vi "SLSC Create Tree Control from EDS datatype.vi"(7 "Property Tree":refnum<vi>, 8 "error in (no error)":errorcluster, 9 "Channel Values":dbl[](array[numeric]), 10 "Properties to enable":string[](array[string]), 11 "SLSC EDS module":T4={"vendorNum"=4660, "vendorName"="National Instruments", "vendorPrefix"="NI", "productNum"=4098, "productName"="SLSC-12201", "capsVersion"="1.0.0a9", "capsSpecVersion"=2, "capsSpecOldestCompatibleVersion"=2, "enums"=[{"name"="NI.Line.Direction", "description-en"="Enumerated values for the direction and output type of a DIO line", "values"=[{"name"="Input", "description-en"="Route line from the front I/O connector to the rear I/O connector", "value"=0}, {"name"="Output_Source", "description-en"="Route line from the rear I/O connector to the front I/O connector with sourcing output topology", "value"=1}, {"name"="Output_Sink", "description-en"="Route line from the rear I/O connector to the front I/O connector with sinking output topology", "value"=2}, {"name"="Output_PushPull", "description-en"="Route line from the rear I/O connector to the front I/O connector with push-pull output topology", "value"=3}]}, {"name"="NI.VsupSource", "description-en"="Enumerated values for the selection of the bank's voltage source", "values"=[{"name"="Vsup_Off", "description-en"="Select neither supply voltage", "value"=0}, {"name"="Vsup_0", "description-en"="Select supply voltage 0", "value"=1}, {"name"="Vsup_1", "description-en"="Select supply voltage 1", "value"=2}]}], "properties"=[{"name"="NI.ModuleControllerVersion", "bitfield"="RevisionReg/DateCode", "value"=variant, "dataType"="UInt32", "min"=variant, "max"=variant, "scale"="", "access"=""}, {"name"="NI.RearBufferState", "bitfield"="RearIOConnectorChannelStateReg/ChannelState", "value"=variant, "dataType"="UInt32", "min"=variant, "max"=variant, "scale"="", "access"=""}, {"name"="NI.FrontBufferState", "bitfield"="FrontIOConnectorChannelStateReg/ChannelState", "value"=variant, "dataType"="UInt32", "min"=variant, "max"=variant, "scale"="", "access"=""}, {"name"="NI.Status24VPowerFailed", "bitfield"="ModuleStatusReg/Status24V_PowerFailed", "value"=variant, "dataType"="Bool", "min"=variant, "max"=variant, "scale"="", "access"=""}, {"name"="NI.Status24VPowerGood", "bitfield"="ModuleStatusReg/Status24V_PowerGood", "value"=variant, "dataType"="Bool", "min"=variant, "max"=variant, "scale"="", "access"=""}, {"name"="NI.Status3_3VPowerGood", "bitfield"="ModuleStatusReg/Status3_3V_PowerGood", "value"=variant, "dataType"="Bool", "min"=variant, "max"=variant, "scale"="", "access"=""}, {"name"="NI.TestModeEnable", "bitfield"="TestModeEnableReg/TestModeEnable", "value"=variant, "dataType"="Bool", "min"=variant, "max"=variant, "scale"="", "access"=""}, {"name"="NI.TestModeValue", "bitfield"="TestModeValueReg/TestModeValue", "value"=variant, "dataType"="UInt32", "min"=variant, "max"=variant, "scale"="", "access"=""}], "commands"=[{"name"="NI.UpdateChannelConfiguration", "description-en"="Command to complete updating physical channel properties", "documentation-en"="This command enables simultaneous updating of the functional state of the module's physical channel configuration. Simultaneous updating of the physical channels' properties prevents the register write commit order from creating unexpected channel configuration states. Run this command to make changes to physical channels' properties take effect.", "startBitfield"="ConfigCommandReg/ChannelConfigurationUpdate", "waitTimeInMs"=5, "doneBitfield"="", "doneInterrupt"="", "doneTimeoutInMs"=0, "value"=variant}, {"name"="NI.UpdateTestMode", "description-en"="Command to complete updating Test Mode properties", "documentation-en"="This command enable simultaneous updating of the functional state of the module's Test Mode configuration. Run this command to make changes to Test Mode properties take effect.", "startBitfield"="ConfigCommandReg/TestModeUpdate", "waitTimeInMs"=0, "doneBitfield"="", "doneInterrupt"="", "doneTimeoutInMs"=0, "value"=variant}, {"name"="NI.Acknowledge24VPowerFailed", "description-en"="Command to acknowledge a latched 24V power failure status", "documentation-en"="This command tries to clear the module's latched true state for the NI.Status24V_PowerFailed property. This command will have no effect on the latched state if the NI.Status24V_PowerGood property is still false.", "startBitfield"="ModuleStatusReg/Status24V_PowerFailedAck", "waitTimeInMs"=0, "doneBitfield"="", "doneInterrupt"="", "doneTimeoutInMs"=0, "value"=variant}], "scales"=[{"name"="InputThreshold33V_Scale", "description-en"="Scales a given voltage into the 10-bit threshold value for the 33V input range", "m"=0.02335, "b"=3.706, "forwardCoeffs"=[], "reverseCoeffs"=[], "coercion"="", "table"=[]}, {"name"="InputThreshold5V_Scale", "description-en"="Scales a given voltage into the 10-bit threshold value for the 5V input range", "m"=0.00441, "b"=0.7, "forwardCoeffs"=[], "reverseCoeffs"=[], "coercion"="", "table"=[]}], "physicalChannels"=[{"name"="bank0", "description-en"="Bank of digital input/output lines on connector J1", "commands"=[], "properties"=[{"name"="NI.VsupSelect", "bitfield"="BankConfigurationReg/Bank0_VsupSelect", "value"=variant, "dataType"="NI.VsupSource", "min"=variant, "max"=variant, "scale"="", "access"=""}, {"name"="NI.RangeEnable5V", "bitfield"="BankConfigurationReg/Bank0_RangeEnable5V", "value"=variant, "dataType"="Bool", "min"=variant, "max"=variant, "scale"="", "access"=""}, {"name"="NI.InputThreshold5V", "bitfield"="BankConfigurationReg/Bank0_InputThreshold5V", "value"=variant, "dataType"="Double", "min"=variant(ext 0.74), "max"=variant(ext 5.1999999999999999998), "scale"="InputThreshold5V_Scale", "access"=""}, {"name"="NI.InputThreshold33V", "bitfield"="BankConfigurationReg/Bank0_InputThreshold33V", "value"=variant, "dataType"="Double", "min"=variant(ext 4.0), "max"=variant(ext 27.7), "scale"="InputThreshold33V_Scale", "access"=""}]}, {"name"="bank1", "description-en"="Bank of digital input/output lines on connector J2", "commands"=[], "properties"=[{"name"="NI.VsupSelect", "bitfield"="BankConfigurationReg/Bank1_VsupSelect", "value"=variant, "dataType"="NI.VsupSource", "min"=variant, "max"=variant, "scale"="", "access"=""}, {"name"="NI.RangeEnable5V", "bitfield"="BankConfigurationReg/Bank1_RangeEnable5V", "value"=variant, "dataType"="Bool", "min"=variant, "max"=variant, "scale"="", "access"=""}, {"name"="NI.InputThreshold5V", "bitfield"="BankConfigurationReg/Bank1_InputThreshold5V", "value"=variant, "dataType"="Double", "min"=variant(ext 0.74), "max"=variant(ext 5.1999999999999999998), "scale"="InputThreshold5V_Scale", "access"=""}, {"name"="NI.InputThreshold33V", "bitfield"="BankConfigurationReg/Bank1_InputThreshold33V", "value"=variant, "dataType"="Double", "min"=variant(ext 4.0), "max"=variant(ext 27.7), "scale"="InputThreshold33V_Scale", "access"=""}]}, {"name"="port0/line0", "description-en"="Configurable digital input/output line with index 0 in bank0.", "commands"=[], "properties"=[{"name"="NI.Line.Index", "bitfield"="", "value"=variant(u64 0), "dataType"="UInt32", "min"=variant, "max"=variant, "scale"="", "access"=""}, {"name"="NI.Line.Direction", "bitfield"="ChannelDirectionReg/Port0_Line0_Direction", "value"=variant, "dataType"="NI.Line.Direction", "min"=variant, "max"=variant, "scale"="", "access"=""}, {"name"="NI.Line.Enable", "bitfield"="ChannelEnableReg/Port0_Line0_Enable", "value"=variant, "dataType"="Bool", "min"=variant, "max"=variant, "scale"="", "access"=""}]}, {"name"="port0/line1", "description-en"="Configurable digital input/output line with index 1 in bank0.", "commands"=[], "properties"=[{"name"="NI.Line.Index", "bitfield"="", "value"=variant(u64 1), "dataType"="UInt32", "min"=variant, "max"=variant, "scale"="", "access"=""}, {"name"="NI.Line.Direction", "bitfield"="ChannelDirectionReg/Port0_Line1_Direction", "value"=variant, "dataType"="NI.Line.Direction", "min"=variant, "max"=variant, "scale"="", "access"=""}, {"name"="NI.Line.Enable", "bitfield"="ChannelEnableReg/Port0_Line1_Enable", "value"=variant, "dataType"="Bool", "min"=variant, "max"=variant, "scale"="", "access"=""}]}, {"name"="port0/line2", "description-en"="Configurable digital input/output line with index 2 in bank0.", "commands"=[], "properties"=[{"name"="NI.Line.Index", "bitfield"="", "value"=variant(u64 2), "dataType"="UInt32", "min"=variant, "max"=variant, "scale"="", "access"=""}, {"name"="NI.Line.Direction", "bitfield"="ChannelDirectionReg/Port0_Line2_Direction", "value"=variant, "dataType"="NI.Line.Direction", "min"=variant, "max"=variant, "scale"="", "access"=""}, {"name"="NI.Line.Enable", "bitfield"="ChannelEnableReg/Port0_Line2_Enable", "value"=variant, "dataType"="Bool", "min"=variant, "max"=variant, "scale"="", "access"=""}]}, {"name"="port0/line3", "description-en"="Configurable digital input/output line with index 3 in bank0.", "commands"=[], "properties"=[{"name"="NI.Line.Index", "bitfield"="", "value"=variant(u64 3), "dataType"="UInt32", "min"=variant, "max"=variant, "scale"="", "access"=""}, {"name"="NI.Line.Direction", "bitfield"="ChannelDirectionReg/Port0_Line3_Direction", "value"=variant, "dataType"="NI.Line.Direction", "min"=variant, "max"=variant, "scale"="", "access"=""}, {"name"="NI.Line.Enable", "bitfield"="ChannelEnableReg/Port0_Line3_Enable", "value"=variant, "dataType"="Bool", "min"=variant, "max"=variant, "scale"="", "access"=""}]}, {"name"="port0/line4", "description-en"="Configurable digital input/output line with index 4 in bank0.", "commands"=[], "properties"=[{"name"="NI.Line.Index", "bitfield"="", "value"=variant(u64 4), "dataType"="UInt32", "min"=variant, "max"=variant, "scale"="", "access"=""}, {"name"="NI.Line.Direction", "bitfield"="ChannelDirectionReg/Port0_Line4_Direction", "value"=variant, "dataType"="NI.Line.Direction", "min"=variant, "max"=variant, "scale"="", "access"=""}, {"name"="NI.Line.Enable", "bitfield"="ChannelEnableReg/Port0_Line4_Enable", "value"=variant, "dataType"="Bool", "min"=variant, "max"=variant, "scale"="", "access"=""}]}, {"name"="port0/line5", "description-en"="Configurable digital input/output line with index 5 in bank0.", "commands"=[], "properties"=[{"name"="NI.Line.Index", "bitfield"="", "value"=variant(u64 5), "dataType"="UInt32", "min"=variant, "max"=variant, "scale"="", "access"=""}, {"name"="NI.Line.Direction", "bitfield"="ChannelDirectionReg/Port0_Line5_Direction", "value"=variant, "dataType"="NI.Line.Direction", "min"=variant, "max"=variant, "scale"="", "access"=""}, {"name"="NI.Line.Enable", "bitfield"="ChannelEnableReg/Port0_Line5_Enable", "value"=variant, "dataType"="Bool", "min"=variant, "max"=variant, "scale"="", "access"=""}]}, {"name"="port0/line6", "description-en"="Configurable digital input/output line with index 6 in bank0.", "commands"=[], "properties"=[{"name"="NI.Line.Index", "bitfield"="", "value"=variant(u64 6), "dataType"="UInt32", "min"=variant, "max"=variant, "scale"="", "access"=""}, {"name"="NI.Line.Direction", "bitfield"="ChannelDirectionReg/Port0_Line6_Direction", "value"=variant, "dataType"="NI.Line.Direction", "min"=variant, "max"=variant, "scale"="", "access"=""}, {"name"="NI.Line.Enable", "bitfield"="ChannelEnableReg/Port0_Line6_Enable", "value"=variant, "dataType"="Bool", "min"=variant, "max"=variant, "scale"="", "access"=""}]}, {"name"="port0/line7", "description-en"="Configurable digital input/output line with index 7 in bank0.", "commands"=[], "properties"=[{"name"="NI.Line.Index", "bitfield"="", "value"=variant(u64 7), "dataType"="UInt32", "min"=variant, "max"=variant, "scale"="", "access"=""}, {"name"="NI.Line.Direction", "bitfield"="ChannelDirectionReg/Port0_Line7_Direction", "value"=variant, "dataType"="NI.Line.Direction", "min"=variant, "max"=variant, "scale"="", "access"=""}, {"name"="NI.Line.Enable", "bitfield"="ChannelEnableReg/Port0_Line7_Enable", "value"=variant, "dataType"="Bool", "min"=variant, "max"=variant, "scale"="", "access"=""}]}, {"name"="port1/line0", "description-en"="Configurable digital input/output line with index 8 in bank0.", "commands"=[], "properties"=[{"name"="NI.Line.Index", "bitfield"="", "value"=variant(u64 8), "dataType"="UInt32", "min"=variant, "max"=variant, "scale"="", "access"=""}, {"name"="NI.Line.Direction", "bitfield"="ChannelDirectionReg/Port1_Line0_Direction", "value"=variant, "dataType"="NI.Line.Direction", "min"=variant, "max"=variant, "scale"="", "access"=""}, {"name"="NI.Line.Enable", "bitfield"="ChannelEnableReg/Port1_Line0_Enable", "value"=variant, "dataType"="Bool", "min"=variant, "max"=variant, "scale"="", "access"=""}]}, {"name"="port1/line1", "description-en"="Configurable digital input/output line with index 9 in bank0.", "commands"=[], "properties"=[{"name"="NI.Line.Index", "bitfield"="", "value"=variant(u64 9), "dataType"="UInt32", "min"=variant, "max"=variant, "scale"="", "access"=""}, {"name"="NI.Line.Direction", "bitfield"="ChannelDirectionReg/Port1_Line1_Direction", "value"=variant, "dataType"="NI.Line.Direction", "min"=variant, "max"=variant, "scale"="", "access"=""}, {"name"="NI.Line.Enable", "bitfield"="ChannelEnableReg/Port1_Line1_Enable", "value"=variant, "dataType"="Bool", "min"=variant, "max"=variant, "scale"="", "access"=""}]}, {"name"="port1/line2", "description-en"="Configurable digital input/output line with index 10 in bank0.", "commands"=[], "properties"=[{"name"="NI.Line.Index", "bitfield"="", "value"=variant(u64 10), "dataType"="UInt32", "min"=variant, "max"=variant, "scale"="", "access"=""}, {"name"="NI.Line.Direction", "bitfield"="ChannelDirectionReg/Port1_Line2_Direction", "value"=variant, "dataType"="NI.Line.Direction", "min"=variant, "max"=variant, "scale"="", "access"=""}, {"name"="NI.Line.Enable", "bitfield"="ChannelEnableReg/Port1_Line2_Enable", "value"=variant, "dataType"="Bool", "min"=variant, "max"=variant, "scale"="", "access"=""}]}, {"name"="port1/line3", "description-en"="Configurable digital input/output line with index 11 in bank0.", "commands"=[], "properties"=[{"name"="NI.Line.Index", "bitfield"="", "value"=variant(u64 11), "dataType"="UInt32", "min"=variant, "max"=variant, "scale"="", "access"=""}, {"name"="NI.Line.Direction", "bitfield"="ChannelDirectionReg/Port1_Line3_Direction", "value"=variant, "dataType"="NI.Line.Direction", "min"=variant, "max"=variant, "scale"="", "access"=""}, {"name"="NI.Line.Enable", "bitfield"="ChannelEnableReg/Port1_Line3_Enable", "value"=variant, "dataType"="Bool", "min"=variant, "max"=variant, "scale"="", "access"=""}]}, {"name"="port1/line4", "description-en"="Configurable digital input/output line with index 12 in bank0.", "commands"=[], "properties"=[{"name"="NI.Line.Index", "bitfield"="", "value"=variant(u64 12), "dataType"="UInt32", "min"=variant, "max"=variant, "scale"="", "access"=""}, {"name"="NI.Line.Direction", "bitfield"="ChannelDirectionReg/Port1_Line4_Direction", "value"=variant, "dataType"="NI.Line.Direction", "min"=variant, "max"=variant, "scale"="", "access"=""}, {"name"="NI.Line.Enable", "bitfield"="ChannelEnableReg/Port1_Line4_Enable", "value"=variant, "dataType"="Bool", "min"=variant, "max"=variant, "scale"="", "access"=""}]}, {"name"="port1/line5", "description-en"="Configurable digital input/output line with index 13 in bank0.", "commands"=[], "properties"=[{"name"="NI.Line.Index", "bitfield"="", "value"=variant(u64 13), "dataType"="UInt32", "min"=variant, "max"=variant, "scale"="", "access"=""}, {"name"="NI.Line.Direction", "bitfield"="ChannelDirectionReg/Port1_Line5_Direction", "value"=variant, "dataType"="NI.Line.Direction", "min"=variant, "max"=variant, "scale"="", "access"=""}, {"name"="NI.Line.Enable", "bitfield"="ChannelEnableReg/Port1_Line5_Enable", "value"=variant, "dataType"="Bool", "min"=variant, "max"=variant, "scale"="", "access"=""}]}, {"name"="port1/line6", "description-en"="Configurable digital input/output line with index 14 in bank0.", "commands"=[], "properties"=[{"name"="NI.Line.Index", "bitfield"="", "value"=variant(u64 14), "dataType"="UInt32", "min"=variant, "max"=variant, "scale"="", "access"=""}, {"name"="NI.Line.Direction", "bitfield"="ChannelDirectionReg/Port1_Line6_Direction", "value"=variant, "dataType"="NI.Line.Direction", "min"=variant, "max"=variant, "scale"="", "access"=""}, {"name"="NI.Line.Enable", "bitfield"="ChannelEnableReg/Port1_Line6_Enable", "value"=variant, "dataType"="Bool", "min"=variant, "max"=variant, "scale"="", "access"=""}]}, {"name"="port1/line7", "description-en"="Configurable digital input/output line with index 15 in bank0.", "commands"=[], "properties"=[{"name"="NI.Line.Index", "bitfield"="", "value"=variant(u64 15), "dataType"="UInt32", "min"=variant, "max"=variant, "scale"="", "access"=""}, {"name"="NI.Line.Direction", "bitfield"="ChannelDirectionReg/Port1_Line7_Direction", "value"=variant, "dataType"="NI.Line.Direction", "min"=variant, "max"=variant, "scale"="", "access"=""}, {"name"="NI.Line.Enable", "bitfield"="ChannelEnableReg/Port1_Line7_Enable", "value"=variant, "dataType"="Bool", "min"=variant, "max"=variant, "scale"="", "access"=""}]}, {"name"="port2/line0", "description-en"="Configurable digital input/output line with index 16 in bank1.", "commands"=[], "properties"=[{"name"="NI.Line.Index", "bitfield"="", "value"=variant(u64 16), "dataType"="UInt32", "min"=variant, "max"=variant, "scale"="", "access"=""}, {"name"="NI.Line.Direction", "bitfield"="ChannelDirectionReg/Port2_Line0_Direction", "value"=variant, "dataType"="NI.Line.Direction", "min"=variant, "max"=variant, "scale"="", "access"=""}, {"name"="NI.Line.Enable", "bitfield"="ChannelEnableReg/Port2_Line0_Enable", "value"=variant, "dataType"="Bool", "min"=variant, "max"=variant, "scale"="", "access"=""}]}, {"name"="port2/line1", "description-en"="Configurable digital input/output line with index 17 in bank1.", "commands"=[], "properties"=[{"name"="NI.Line.Index", "bitfield"="", "value"=variant(u64 17), "dataType"="UInt32", "min"=variant, "max"=variant, "scale"="", "access"=""}, {"name"="NI.Line.Direction", "bitfield"="ChannelDirectionReg/Port2_Line1_Direction", "value"=variant, "dataType"="NI.Line.Direction", "min"=variant, "max"=variant, "scale"="", "access"=""}, {"name"="NI.Line.Enable", "bitfield"="ChannelEnableReg/Port2_Line1_Enable", "value"=variant, "dataType"="Bool", "min"=variant, "max"=variant, "scale"="", "access"=""}]}, {"name"="port2/line2", "description-en"="Configurable digital input/output line with index 18 in bank1.", "commands"=[], "properties"=[{"name"="NI.Line.Index", "bitfield"="", "value"=variant(u64 18), "dataType"="UInt32", "min"=variant, "max"=variant, "scale"="", "access"=""}, {"name"="NI.Line.Direction", "bitfield"="ChannelDirectionReg/Port2_Line2_Direction", "value"=variant, "dataType"="NI.Line.Direction", "min"=variant, "max"=variant, "scale"="", "access"=""}, {"name"="NI.Line.Enable", "bitfield"="ChannelEnableReg/Port2_Line2_Enable", "value"=variant, "dataType"="Bool", "min"=variant, "max"=variant, "scale"="", "access"=""}]}, {"name"="port2/line3", "description-en"="Configurable digital input/output line with index 19 in bank1.", "commands"=[], "properties"=[{"name"="NI.Line.Index", "bitfield"="", "value"=variant(u64 19), "dataType"="UInt32", "min"=variant, "max"=variant, "scale"="", "access"=""}, {"name"="NI.Line.Direction", "bitfield"="ChannelDirectionReg/Port2_Line3_Direction", "value"=variant, "dataType"="NI.Line.Direction", "min"=variant, "max"=variant, "scale"="", "access"=""}, {"name"="NI.Line.Enable", "bitfield"="ChannelEnableReg/Port2_Line3_Enable", "value"=variant, "dataType"="Bool", "min"=variant, "max"=variant, "scale"="", "access"=""}]}, {"name"="port2/line4", "description-en"="Configurable digital input/output line with index 20 in bank1.", "commands"=[], "properties"=[{"name"="NI.Line.Index", "bitfield"="", "value"=variant(u64 20), "dataType"="UInt32", "min"=variant, "max"=variant, "scale"="", "access"=""}, {"name"="NI.Line.Direction", "bitfield"="ChannelDirectionReg/Port2_Line4_Direction", "value"=variant, "dataType"="NI.Line.Direction", "min"=variant, "max"=variant, "scale"="", "access"=""}, {"name"="NI.Line.Enable", "bitfield"="ChannelEnableReg/Port2_Line4_Enable", "value"=variant, "dataType"="Bool", "min"=variant, "max"=variant, "scale"="", "access"=""}]}, {"name"="port2/line5", "description-en"="Configurable digital input/output line with index 21 in bank1.", "commands"=[], "properties"=[{"name"="NI.Line.Index", "bitfield"="", "value"=variant(u64 21), "dataType"="UInt32", "min"=variant, "max"=variant, "scale"="", "access"=""}, {"name"="NI.Line.Direction", "bitfield"="ChannelDirectionReg/Port2_Line5_Direction", "value"=variant, "dataType"="NI.Line.Direction", "min"=variant, "max"=variant, "scale"="", "access"=""}, {"name"="NI.Line.Enable", "bitfield"="ChannelEnableReg/Port2_Line5_Enable", "value"=variant, "dataType"="Bool", "min"=variant, "max"=variant, "scale"="", "access"=""}]}, {"name"="port2/line6", "description-en"="Configurable digital input/output line with index 22 in bank1.", "commands"=[], "properties"=[{"name"="NI.Line.Index", "bitfield"="", "value"=variant(u64 22), "dataType"="UInt32", "min"=variant, "max"=variant, "scale"="", "access"=""}, {"name"="NI.Line.Direction", "bitfield"="ChannelDirectionReg/Port2_Line6_Direction", "value"=variant, "dataType"="NI.Line.Direction", "min"=variant, "max"=variant, "scale"="", "access"=""}, {"name"="NI.Line.Enable", "bitfield"="ChannelEnableReg/Port2_Line6_Enable", "value"=variant, "dataType"="Bool", "min"=variant, "max"=variant, "scale"="", "access"=""}]}, {"name"="port2/line7", "description-en"="Configurable digital input/output line with index 23 in bank1.", "commands"=[], "properties"=[{"name"="NI.Line.Index", "bitfield"="", "value"=variant(u64 23), "dataType"="UInt32", "min"=variant, "max"=variant, "scale"="", "access"=""}, {"name"="NI.Line.Direction", "bitfield"="ChannelDirectionReg/Port2_Line7_Direction", "value"=variant, "dataType"="NI.Line.Direction", "min"=variant, "max"=variant, "scale"="", "access"=""}, {"name"="NI.Line.Enable", "bitfield"="ChannelEnableReg/Port2_Line7_Enable", "value"=variant, "dataType"="Bool", "min"=variant, "max"=variant, "scale"="", "access"=""}]}, {"name"="port3/line0", "description-en"="Configurable digital input/output line with index 24 in bank1.", "commands"=[], "properties"=[{"name"="NI.Line.Index", "bitfield"="", "value"=variant(u64 24), "dataType"="UInt32", "min"=variant, "max"=variant, "scale"="", "access"=""}, {"name"="NI.Line.Direction", "bitfield"="ChannelDirectionReg/Port3_Line0_Direction", "value"=variant, "dataType"="NI.Line.Direction", "min"=variant, "max"=variant, "scale"="", "access"=""}, {"name"="NI.Line.Enable", "bitfield"="ChannelEnableReg/Port3_Line0_Enable", "value"=variant, "dataType"="Bool", "min"=variant, "max"=variant, "scale"="", "access"=""}]}, {"name"="port3/line1", "description-en"="Configurable digital input/output line with index 25 in bank1.", "commands"=[], "properties"=[{"name"="NI.Line.Index", "bitfield"="", "value"=variant(u64 25), "dataType"="UInt32", "min"=variant, "max"=variant, "scale"="", "access"=""}, {"name"="NI.Line.Direction", "bitfield"="ChannelDirectionReg/Port3_Line1_Direction", "value"=variant, "dataType"="NI.Line.Direction", "min"=variant, "max"=variant, "scale"="", "access"=""}, {"name"="NI.Line.Enable", "bitfield"="ChannelEnableReg/Port3_Line1_Enable", "value"=variant, "dataType"="Bool", "min"=variant, "max"=variant, "scale"="", "access"=""}]}, {"name"="port3/line2", "description-en"="Configurable digital input/output line with index 26 in bank1.", "commands"=[], "properties"=[{"name"="NI.Line.Index", "bitfield"="", "value"=variant(u64 26), "dataType"="UInt32", "min"=variant, "max"=variant, "scale"="", "access"=""}, {"name"="NI.Line.Direction", "bitfield"="ChannelDirectionReg/Port3_Line2_Direction", "value"=variant, "dataType"="NI.Line.Direction", "min"=variant, "max"=variant, "scale"="", "access"=""}, {"name"="NI.Line.Enable", "bitfield"="ChannelEnableReg/Port3_Line2_Enable", "value"=variant, "dataType"="Bool", "min"=variant, "max"=variant, "scale"="", "access"=""}]}, {"name"="port3/line3", "description-en"="Configurable digital input/output line with index 27 in bank1.", "commands"=[], "properties"=[{"name"="NI.Line.Index", "bitfield"="", "value"=variant(u64 27), "dataType"="UInt32", "min"=variant, "max"=variant, "scale"="", "access"=""}, {"name"="NI.Line.Direction", "bitfield"="ChannelDirectionReg/Port3_Line3_Direction", "value"=variant, "dataType"="NI.Line.Direction", "min"=variant, "max"=variant, "scale"="", "access"=""}, {"name"="NI.Line.Enable", "bitfield"="ChannelEnableReg/Port3_Line3_Enable", "value"=variant, "dataType"="Bool", "min"=variant, "max"=variant, "scale"="", "access"=""}]}, {"name"="port3/line4", "description-en"="Configurable digital input/output line with index 28 in bank1.", "commands"=[], "properties"=[{"name"="NI.Line.Index", "bitfield"="", "value"=variant(u64 28), "dataType"="UInt32", "min"=variant, "max"=variant, "scale"="", "access"=""}, {"name"="NI.Line.Direction", "bitfield"="ChannelDirectionReg/Port3_Line4_Direction", "value"=variant, "dataType"="NI.Line.Direction", "min"=variant, "max"=variant, "scale"="", "access"=""}, {"name"="NI.Line.Enable", "bitfield"="ChannelEnableReg/Port3_Line4_Enable", "value"=variant, "dataType"="Bool", "min"=variant, "max"=variant, "scale"="", "access"=""}]}, {"name"="port3/line5", "description-en"="Configurable digital input/output line with index 29 in bank1.", "commands"=[], "properties"=[{"name"="NI.Line.Index", "bitfield"="", "value"=variant(u64 29), "dataType"="UInt32", "min"=variant, "max"=variant, "scale"="", "access"=""}, {"name"="NI.Line.Direction", "bitfield"="ChannelDirectionReg/Port3_Line5_Direction", "value"=variant, "dataType"="NI.Line.Direction", "min"=variant, "max"=variant, "scale"="", "access"=""}, {"name"="NI.Line.Enable", "bitfield"="ChannelEnableReg/Port3_Line5_Enable", "value"=variant, "dataType"="Bool", "min"=variant, "max"=variant, "scale"="", "access"=""}]}, {"name"="port3/line6", "description-en"="Configurable digital input/output line with index 30 in bank1.", "commands"=[], "properties"=[{"name"="NI.Line.Index", "bitfield"="", "value"=variant(u64 30), "dataType"="UInt32", "min"=variant, "max"=variant, "scale"="", "access"=""}, {"name"="NI.Line.Direction", "bitfield"="ChannelDirectionReg/Port3_Line6_Direction", "value"=variant, "dataType"="NI.Line.Direction", "min"=variant, "max"=variant, "scale"="", "access"=""}, {"name"="NI.Line.Enable", "bitfield"="ChannelEnableReg/Port3_Line6_Enable", "value"=variant, "dataType"="Bool", "min"=variant, "max"=variant, "scale"="", "access"=""}]}, {"name"="port3/line7", "description-en"="Configurable digital input/output line with index 31 in bank1.", "commands"=[], "properties"=[{"name"="NI.Line.Index", "bitfield"="", "value"=variant(u64 31), "dataType"="UInt32", "min"=variant, "max"=variant, "scale"="", "access"=""}, {"name"="NI.Line.Direction", "bitfield"="ChannelDirectionReg/Port3_Line7_Direction", "value"=variant, "dataType"="NI.Line.Direction", "min"=variant, "max"=variant, "scale"="", "access"=""}, {"name"="NI.Line.Enable", "bitfield"="ChannelEnableReg/Port3_Line7_Enable", "value"=variant, "dataType"="Bool", "min"=variant, "max"=variant, "scale"="", "access"=""}]}], "registerMap"={"registers"=[{"name"="RevisionReg", "description-en"="Register for the DateCode", "access"="ReadOnly", "address"=0, "size"=32, "bitfields"=[{"name"="DateCode", "description-en"="CPLD revision date code", "offset"=0, "size"=32, "signed"=FALSE, "strobe"=FALSE}]}, {"name"="RearIOConnectorChannelStateReg", "description-en"="Register for the rear I/O connector channel state", "access"="ReadOnly", "address"=4, "size"=32, "bitfields"=[{"name"="ChannelState", "description-en"="Logic state of all rear I/O connector input buffers", "offset"=0, "size"=32, "signed"=FALSE, "strobe"=FALSE}]}, {"name"="FrontIOConnectorChannelStateReg", "description-en"="Register for the front I/O connector channel state", "access"="ReadOnly", "address"=8, "size"=32, "bitfields"=[{"name"="ChannelState", "description-en"="Logic state of all front I/O connector input buffers", "offset"=0, "size"=32, "signed"=FALSE, "strobe"=FALSE}]}, {"name"="ModuleStatusReg", "description-en"="Register for monitoring board-level module status", "access"="ReadWrite", "address"=12, "size"=8, "bitfields"=[{"name"="Status3_3V_PowerGood", "description-en"="3.3V power status (always '1' on successful module access)", "offset"=0, "size"=1, "signed"=FALSE, "strobe"=FALSE}, {"name"="Status24V_PowerGood", "description-en"="24V power status", "offset"=1, "size"=1, "signed"=FALSE, "strobe"=FALSE}, {"name"="Status24V_PowerFailed", "description-en"="Latching status indicating 24V power failure", "offset"=2, "size"=1, "signed"=FALSE, "strobe"=FALSE}, {"name"="Status24V_PowerFailedAck", "description-en"="Target bitfield for the NI.Status24V_PowerFailedAck command", "offset"=3, "size"=1, "signed"=FALSE, "strobe"=TRUE}]}, {"name"="ChannelDirectionReg", "description-en"="Register for setting channel direction (This register requires having a valid \"initalValue\" set.)", "access"="ReadWrite", "address"=64, "size"=64, "bitfields"=[{"name"="Port0_Line0_Direction", "description-en"="", "offset"=0, "size"=2, "signed"=FALSE, "strobe"=FALSE}, {"name"="Port0_Line1_Direction", "description-en"="", "offset"=2, "size"=2, "signed"=FALSE, "strobe"=FALSE}, {"name"="Port0_Line2_Direction", "description-en"="", "offset"=4, "size"=2, "signed"=FALSE, "strobe"=FALSE}, {"name"="Port0_Line3_Direction", "description-en"="", "offset"=6, "size"=2, "signed"=FALSE, "strobe"=FALSE}, {"name"="Port0_Line4_Direction", "description-en"="", "offset"=8, "size"=2, "signed"=FALSE, "strobe"=FALSE}, {"name"="Port0_Line5_Direction", "description-en"="", "offset"=10, "size"=2, "signed"=FALSE, "strobe"=FALSE}, {"name"="Port0_Line6_Direction", "description-en"="", "offset"=12, "size"=2, "signed"=FALSE, "strobe"=FALSE}, {"name"="Port0_Line7_Direction", "description-en"="", "offset"=14, "size"=2, "signed"=FALSE, "strobe"=FALSE}, {"name"="Port1_Line0_Direction", "description-en"="", "offset"=16, "size"=2, "signed"=FALSE, "strobe"=FALSE}, {"name"="Port1_Line1_Direction", "description-en"="", "offset"=18, "size"=2, "signed"=FALSE, "strobe"=FALSE}, {"name"="Port1_Line2_Direction", "description-en"="", "offset"=20, "size"=2, "signed"=FALSE, "strobe"=FALSE}, {"name"="Port1_Line3_Direction", "description-en"="", "offset"=22, "size"=2, "signed"=FALSE, "strobe"=FALSE}, {"name"="Port1_Line4_Direction", "description-en"="", "offset"=24, "size"=2, "signed"=FALSE, "strobe"=FALSE}, {"name"="Port1_Line5_Direction", "description-en"="", "offset"=26, "size"=2, "signed"=FALSE, "strobe"=FALSE}, {"name"="Port1_Line6_Direction", "description-en"="", "offset"=28, "size"=2, "signed"=FALSE, "strobe"=FALSE}, {"name"="Port1_Line7_Direction", "description-en"="", "offset"=30, "size"=2, "signed"=FALSE, "strobe"=FALSE}, {"name"="Port2_Line0_Direction", "description-en"="", "offset"=32, "size"=2, "signed"=FALSE, "strobe"=FALSE}, {"name"="Port2_Line1_Direction", "description-en"="", "offset"=34, "size"=2, "signed"=FALSE, "strobe"=FALSE}, {"name"="Port2_Line2_Direction", "description-en"="", "offset"=36, "size"=2, "signed"=FALSE, "strobe"=FALSE}, {"name"="Port2_Line3_Direction", "description-en"="", "offset"=38, "size"=2, "signed"=FALSE, "strobe"=FALSE}, {"name"="Port2_Line4_Direction", "description-en"="", "offset"=40, "size"=2, "signed"=FALSE, "strobe"=FALSE}, {"name"="Port2_Line5_Direction", "description-en"="", "offset"=42, "size"=2, "signed"=FALSE, "strobe"=FALSE}, {"name"="Port2_Line6_Direction", "description-en"="", "offset"=44, "size"=2, "signed"=FALSE, "strobe"=FALSE}, {"name"="Port2_Line7_Direction", "description-en"="", "offset"=46, "size"=2, "signed"=FALSE, "strobe"=FALSE}, {"name"="Port3_Line0_Direction", "description-en"="", "offset"=48, "size"=2, "signed"=FALSE, "strobe"=FALSE}, {"name"="Port3_Line1_Direction", "description-en"="", "offset"=50, "size"=2, "signed"=FALSE, "strobe"=FALSE}, {"name"="Port3_Line2_Direction", "description-en"="", "offset"=52, "size"=2, "signed"=FALSE, "strobe"=FALSE}, {"name"="Port3_Line3_Direction", "description-en"="", "offset"=54, "size"=2, "signed"=FALSE, "strobe"=FALSE}, {"name"="Port3_Line4_Direction", "description-en"="", "offset"=56, "size"=2, "signed"=FALSE, "strobe"=FALSE}, {"name"="Port3_Line5_Direction", "description-en"="", "offset"=58, "size"=2, "signed"=FALSE, "strobe"=FALSE}, {"name"="Port3_Line6_Direction", "description-en"="", "offset"=60, "size"=2, "signed"=FALSE, "strobe"=FALSE}, {"name"="Port3_Line7_Direction", "description-en"="", "offset"=62, "size"=2, "signed"=FALSE, "strobe"=FALSE}]}, {"name"="ChannelEnableReg", "description-en"="Register for setting channel enable (This register requires having a valid \"initalValue\" set.)", "access"="ReadWrite", "address"=72, "size"=32, "bitfields"=[{"name"="Port0_Line0_Enable", "description-en"="", "offset"=0, "size"=1, "signed"=FALSE, "strobe"=FALSE}, {"name"="Port0_Line1_Enable", "description-en"="", "offset"=1, "size"=1, "signed"=FALSE, "strobe"=FALSE}, {"name"="Port0_Line2_Enable", "description-en"="", "offset"=2, "size"=1, "signed"=FALSE, "strobe"=FALSE}, {"name"="Port0_Line3_Enable", "description-en"="", "offset"=3, "size"=1, "signed"=FALSE, "strobe"=FALSE}, {"name"="Port0_Line4_Enable", "description-en"="", "offset"=4, "size"=1, "signed"=FALSE, "strobe"=FALSE}, {"name"="Port0_Line5_Enable", "description-en"="", "offset"=5, "size"=1, "signed"=FALSE, "strobe"=FALSE}, {"name"="Port0_Line6_Enable", "description-en"="", "offset"=6, "size"=1, "signed"=FALSE, "strobe"=FALSE}, {"name"="Port0_Line7_Enable", "description-en"="", "offset"=7, "size"=1, "signed"=FALSE, "strobe"=FALSE}, {"name"="Port1_Line0_Enable", "description-en"="", "offset"=8, "size"=1, "signed"=FALSE, "strobe"=FALSE}, {"name"="Port1_Line1_Enable", "description-en"="", "offset"=9, "size"=1, "signed"=FALSE, "strobe"=FALSE}, {"name"="Port1_Line2_Enable", "description-en"="", "offset"=10, "size"=1, "signed"=FALSE, "strobe"=FALSE}, {"name"="Port1_Line3_Enable", "description-en"="", "offset"=11, "size"=1, "signed"=FALSE, "strobe"=FALSE}, {"name"="Port1_Line4_Enable", "description-en"="", "offset"=12, "size"=1, "signed"=FALSE, "strobe"=FALSE}, {"name"="Port1_Line5_Enable", "description-en"="", "offset"=13, "size"=1, "signed"=FALSE, "strobe"=FALSE}, {"name"="Port1_Line6_Enable", "description-en"="", "offset"=14, "size"=1, "signed"=FALSE, "strobe"=FALSE}, {"name"="Port1_Line7_Enable", "description-en"="", "offset"=15, "size"=1, "signed"=FALSE, "strobe"=FALSE}, {"name"="Port2_Line0_Enable", "description-en"="", "offset"=16, "size"=1, "signed"=FALSE, "strobe"=FALSE}, {"name"="Port2_Line1_Enable", "description-en"="", "offset"=17, "size"=1, "signed"=FALSE, "strobe"=FALSE}, {"name"="Port2_Line2_Enable", "description-en"="", "offset"=18, "size"=1, "signed"=FALSE, "strobe"=FALSE}, {"name"="Port2_Line3_Enable", "description-en"="", "offset"=19, "size"=1, "signed"=FALSE, "strobe"=FALSE}, {"name"="Port2_Line4_Enable", "description-en"="", "offset"=20, "size"=1, "signed"=FALSE, "strobe"=FALSE}, {"name"="Port2_Line5_Enable", "description-en"="", "offset"=21, "size"=1, "signed"=FALSE, "strobe"=FALSE}, {"name"="Port2_Line6_Enable", "description-en"="", "offset"=22, "size"=1, "signed"=FALSE, "strobe"=FALSE}, {"name"="Port2_Line7_Enable", "description-en"="", "offset"=23, "size"=1, "signed"=FALSE, "strobe"=FALSE}, {"name"="Port3_Line0_Enable", "description-en"="", "offset"=24, "size"=1, "signed"=FALSE, "strobe"=FALSE}, {"name"="Port3_Line1_Enable", "description-en"="", "offset"=25, "size"=1, "signed"=FALSE, "strobe"=FALSE}, {"name"="Port3_Line2_Enable", "description-en"="", "offset"=26, "size"=1, "signed"=FALSE, "strobe"=FALSE}, {"name"="Port3_Line3_Enable", "description-en"="", "offset"=27, "size"=1, "signed"=FALSE, "strobe"=FALSE}, {"name"="Port3_Line4_Enable", "description-en"="", "offset"=28, "size"=1, "signed"=FALSE, "strobe"=FALSE}, {"name"="Port3_Line5_Enable", "description-en"="", "offset"=29, "size"=1, "signed"=FALSE, "strobe"=FALSE}, {"name"="Port3_Line6_Enable", "description-en"="", "offset"=30, "size"=1, "signed"=FALSE, "strobe"=FALSE}, {"name"="Port3_Line7_Enable", "description-en"="", "offset"=31, "size"=1, "signed"=FALSE, "strobe"=FALSE}]}, {"name"="BankConfigurationReg", "description-en"="Register for configuring bank settings (This register requires having a valid \"initalValue\" set.)", "access"="ReadWrite", "address"=76, "size"=64, "bitfields"=[{"name"="Bank0_VsupSelect", "description-en"="", "offset"=0, "size"=2, "signed"=FALSE, "strobe"=FALSE}, {"name"="Bank0_RangeEnable5V", "description-en"="", "offset"=2, "size"=1, "signed"=FALSE, "strobe"=FALSE}, {"name"="Bank0_InputThreshold5V", "description-en"="", "offset"=4, "size"=10, "signed"=FALSE, "strobe"=FALSE}, {"name"="Bank0_InputThreshold33V", "description-en"="", "offset"=16, "size"=10, "signed"=FALSE, "strobe"=FALSE}, {"name"="Bank1_VsupSelect", "description-en"="", "offset"=32, "size"=2, "signed"=FALSE, "strobe"=FALSE}, {"name"="Bank1_RangeEnable5V", "description-en"="", "offset"=34, "size"=1, "signed"=FALSE, "strobe"=FALSE}, {"name"="Bank1_InputThreshold5V", "description-en"="", "offset"=36, "size"=10, "signed"=FALSE, "strobe"=FALSE}, {"name"="Bank1_InputThreshold33V", "description-en"="", "offset"=48, "size"=10, "signed"=FALSE, "strobe"=FALSE}]}, {"name"="TestModeEnableReg", "description-en"="Register for setting Test Mode enable (This register requires having a valid \"initalValue\" set.)", "access"="ReadWrite", "address"=84, "size"=8, "bitfields"=[{"name"="TestModeEnable", "description-en"="", "offset"=0, "size"=1, "signed"=FALSE, "strobe"=FALSE}]}, {"name"="TestModeValueReg", "description-en"="Register for setting Test Mode value (This register requires having a valid \"initalValue\" set.)", "access"="ReadWrite", "address"=88, "size"=32, "bitfields"=[{"name"="TestModeValue", "description-en"="", "offset"=0, "size"=32, "signed"=FALSE, "strobe"=FALSE}]}, {"name"="ConfigCommandReg", "description-en"="Register for configuration update commands", "access"="ReadWrite", "address"=92, "size"=8, "bitfields"=[{"name"="ChannelConfigurationUpdate", "description-en"="Target bitfield for the NI.ChannelConfigurationUpdate command", "offset"=0, "size"=1, "signed"=FALSE, "strobe"=TRUE}, {"name"="TestModeUpdate", "description-en"="Target bitfield for the NI.TestModeUpdate command", "offset"=1, "size"=1, "signed"=FALSE, "strobe"=TRUE}]}, {"name"="ReservedConfigReg", "description-en"="Reserved configuration register. Do not modify the value stored in this register. Do not set an \"initialValue\" on this register.", "access"="ReadWrite", "address"=96, "size"=8, "bitfields"=[{"name"="Reserved", "description-en"="", "offset"=0, "size"=4, "signed"=FALSE, "strobe"=FALSE}]}, {"name"="ComplianceTestReg", "description-en"="SLSC Predefined Register: Compliance Test Register", "access"="ReadWrite", "address"=32512, "size"=8, "bitfields"=[{"name"="Scratch", "description-en"="8-bit value storage", "offset"=0, "size"=8, "signed"=FALSE, "strobe"=FALSE}]}, {"name"="ComplianceTestPatternReg", "description-en"="SLSC Predefined Register: Compliance Test Pattern Register", "access"="ReadOnly", "address"=32520, "size"=64, "bitfields"=[{"name"="Pattern", "description-en"="Test pattern with fixed value 0xAA55F733CC08D24B", "offset"=0, "size"=64, "signed"=FALSE, "strobe"=FALSE}]}]}}) -> (0 "error out":errorcluster, 1 "Enum Strings":cluster{"name":string, string}[](array[cluster]), 2 "Enums":T1[](array[typedef]), 3 "SLSC Output Tree":T3(array[cluster])=[{"Left Cell String"="SLSC-12001-030EE1BC-Mod8", "Child Text"=[], "Child Tag"="Device", "Item Indent"=0, "Child Only?"=FALSE, "Glyph Index"=28}, {"Left Cell String"="Commands", "Child Text"=[], "Child Tag"="Device/Commands", "Item Indent"=1, "Child Only?"=FALSE, "Glyph Index"=35}, {"Left Cell String"="NI.UpdateChannelConfiguration", "Child Text"=["", "", "", "", "", "", "Command..NI.UpdateChannelConfiguration", "Command to complete updating physical channel properties", "This command enables simultaneous updating of the functional state of the module's physical channel configuration. Simultaneous updating of the physical channels' properties prevents the register write commit order from creating unexpected channel configuration states. Run this command to make changes to physical channels' properties take effect."], "Child Tag"="Device/Commands/NI.UpdateChannelConfiguration", "Item Indent"=2, "Child Only?"=FALSE, "Glyph Index"=4}, {"Left Cell String"="NI.UpdateTestMode", "Child Text"=["", "", "", "", "", "", "Command..NI.UpdateTestMode", "Command to complete updating Test Mode properties", "This command enable simultaneous updating of the functional state of the module's Test Mode configuration. Run this command to make changes to Test Mode properties take effect."], "Child Tag"="Device/Commands/NI.UpdateTestMode", "Item Indent"=2, "Child Only?"=FALSE, "Glyph Index"=4}, {"Left Cell String"="NI.Acknowledge24VPowerFailed", "Child Text"=["", "", "", "", "", "", "Command..NI.Acknowledge24VPowerFailed", "Command to acknowledge a latched 24V power failure status", "This command tries to clear the module's latched true state for the NI.Status24V_PowerFailed property. This command will have no effect on the latched state if the NI.Status24V_PowerGood property is still false."], "Child Tag"="Device/Commands/NI.Acknowledge24VPowerFailed", "Item Indent"=2, "Child Only?"=FALSE, "Glyph Index"=4}, {"Left Cell String"="Properties", "Child Text"=[], "Child Tag"="Device/Properties", "Item Indent"=1, "Child Only?"=FALSE, "Glyph Index"=36}, {"Left Cell String"="NI.ModuleControllerVersion", "Child Text"=["17022812", "Read Only", "U32", "", "", "", "[3.860173E+8].R.U32..NI.ModuleControllerVersion", "Module Controller Version", "The version is the timestamp, in hexadecimal format, of the time the Module Controller was compiled."], "Child Tag"="Device/Properties/NI.ModuleControllerVersion", "Item Indent"=2, "Child Only?"=FALSE, "Glyph Index"=8}, {"Left Cell String"="NI.RearBufferState", "Child Text"=["0", "Read Only", "U32", "", "", "", "[0].R.U32..NI.RearBufferState", "Logic state of all rear I/O connector input buffers", "Reading this property retrieves the current logic state of the rear I/O connector input buffers. This retrieval is controlled through the software system so the actual sampling time of the inputs is not deterministic. The value at each bit position is a function of the logic state at the XJ2 pin and the corresponding line's direction and enable configuration. An enabled line configured as an input will drive the rear I/O connector input buffer to the same state as detected at the front I/O connector input buffer."], "Child Tag"="Device/Properties/NI.RearBufferState", "Item Indent"=2, "Child Only?"=FALSE, "Glyph Index"=8}, {"Left Cell String"="NI.FrontBufferState", "Child Text"=["0", "Read Only", "U32", "", "", "", "[0].R.U32..NI.FrontBufferState", "Logic state of all front I/O connector input buffers", "Reading this property retrieves the current logic state of the front I/O connector input buffers. This retrieval is controlled through the software system so the actual sampling time of the inputs is not deterministic. The value at each bit position is a function of the voltage at the module DSUB pin and the bank range and threshold configuration. An enabled line configured as an output may drive the front I/O connector input buffer to a specific voltage, depending on the bank supply voltage configuration, the line's output topology, and the line's logic state from the rear I/O connector input buffer."], "Child Tag"="Device/Properties/NI.FrontBufferState", "Item Indent"=2, "Child Only?"=FALSE, "Glyph Index"=8}, {"Left Cell String"="NI.Status24VPowerFailed", "Child Text"=["False", "Read Only", "Bool", "", "", "", "[0].R.Bool..NI.Status24VPowerFailed", "State of the latched failure status of the module's 24V rail from the SLSC Interface", "When the NI.Status24V_PowerGood becomes false, this property latches as true until it is reset by the NI.Status24V_FaultAcknowledge command is sent after NI.Status24V_PowerGood returns to true. If this property is true, then the supply voltage selection for both banks of the module has been forced off for a nonzero duration."], "Child Tag"="Device/Properties/NI.Status24VPowerFailed", "Item Indent"=2, "Child Only?"=FALSE, "Glyph Index"=8}, {"Left Cell String"="NI.Status24VPowerGood", "Child Text"=["True", "Read Only", "Bool", "", "", "", "[1].R.Bool..NI.Status24VPowerGood", "State of the 24V rail on the module from the SLSC Interface", "When the 24V rail from the SLSC Interface drops below the safe operating range for the module, this property is set to false. Simultaneously, to protect the module's output circuitry and to prevent the module front I/O connector outputs from glitching high, the supply voltage selection for both banks is forced off until the 24V rail recovers and is stable."], "Child Tag"="Device/Properties/NI.Status24VPowerGood", "Item Indent"=2, "Child Only?"=FALSE, "Glyph Index"=8}, {"Left Cell String"="NI.Status3_3VPowerGood", "Child Text"=["True", "Read Only", "Bool", "", "", "", "[1].R.Bool..NI.Status3_3VPowerGood", "State of the 3.3V rail from the SLSC Interface on the module", "This property will always be true on a correctly functioning module because the module CPLD requires the 3.3V rail from the SLSC Interface to operate."], "Child Tag"="Device/Properties/NI.Status3_3VPowerGood", "Item Indent"=2, "Child Only?"=FALSE, "Glyph Index"=8}, {"Left Cell String"="NI.TestModeEnable", "Child Text"=["False", "Read/Write", "Bool", "", "", "", "[0].RW.Bool..NI.TestModeEnable", "Enable for Test Mode", "Enable state for the module's Test Mode. When Test Mode is enabled, the module will output the values from the NI.TestModeValue property on the corresponding lines. Each line's respective direction and enable configuration will still apply when Test Mode is active. The data source of the lines is the only change when Test Mode is active. Changes to this property take effect after running the NI.TestModeUpdate command."], "Child Tag"="Device/Properties/NI.TestModeEnable", "Item Indent"=2, "Child Only?"=FALSE, "Glyph Index"=9}, {"Left Cell String"="NI.TestModeValue", "Child Text"=["0", "Read/Write", "U32", "", "", "", "[0].RW.U32..NI.TestModeValue", "Output logic states for use during Test Mode", "Output logic states for the module for use during Test Mode. The logic state corresponding to each line may be set independently of the other states. Changes to this property take effect after running the NI.TestModeUpdate command."], "Child Tag"="Device/Properties/NI.TestModeValue", "Item Indent"=2, "Child Only?"=FALSE, "Glyph Index"=9}, {"Left Cell String"="SLSC-12001-030EE1BC-Mod8/bank0", "Child Text"=[], "Child Tag"="Physical Channel/bank0", "Item Indent"=1, "Child Only?"=FALSE, "Glyph Index"=31}, {"Left Cell String"="Commands", "Child Text"=[], "Child Tag"="Physical Channel/bank0/Commands", "Item Indent"=2, "Child Only?"=FALSE, "Glyph Index"=35}, {"Left Cell String"="Properties", "Child Text"=[], "Child Tag"="Physical Channel/bank0/Properties", "Item Indent"=2, "Child Only?"=FALSE, "Glyph Index"=36}, {"Left Cell String"="NI.VsupSelect", "Child Text"=["[0]Vsup_Off", "Read/Write", "I32", "Enum", "NI.VsupSource", "[0]Vsup_Off;[1]Vsup_0;[2]Vsup_1;", "[0].RW.I32.bank0.NI.VsupSelect", "Voltage source selection", "Voltage source selection for this bank. Changes to this property take effect after running the NI.ChannelConfigurationUpdate command."], "Child Tag"="Physical Channel/bank0/Properties/NI.VsupSelect", "Item Indent"=3, "Child Only?"=FALSE, "Glyph Index"=9}, {"Left Cell String"="NI.RangeEnable5V", "Child Text"=["False", "Read/Write", "Bool", "", "", "", "[0].RW.Bool.bank0.NI.RangeEnable5V", "Voltage range selection", "Enable state for this bank's voltage range. When enabled, this bank uses the NI.InputThreshold5V for the input threshold. When disabled, this bank uses the NI.InputThreshold33V for the input threshold. Changes to this property take effect after running the NI.ChannelConfigurationUpdate command."], "Child Tag"="Physical Channel/bank0/Properties/NI.RangeEnable5V", "Item Indent"=3, "Child Only?"=FALSE, "Glyph Index"=9}, {"Left Cell String"="NI.InputThreshold5V", "Child Text"=["0.7", "Read/Write", "DBL", "", "", "", "[0.7].RW.DBL.bank0.NI.InputThreshold5V", "Input threshold voltage for the 5 V range", "Input threshold voltage for this bank when its NI.RangeEnable5V is true. Changes to this property take effect after running the NI.ChannelConfigurationUpdate command."], "Child Tag"="Physical Channel/bank0/Properties/NI.InputThreshold5V", "Item Indent"=3, "Child Only?"=FALSE, "Glyph Index"=9}, {"Left Cell String"="NI.InputThreshold33V", "Child Text"=["3.706", "Read/Write", "DBL", "", "", "", "[3.706].RW.DBL.bank0.NI.InputThreshold33V", "Input threshold voltage for the 33 V range", "Input threshold voltage for this bank when its NI.RangeEnable5V is false. Changes to this property take effect after running the NI.ChannelConfigurationUpdate command."], "Child Tag"="Physical Channel/bank0/Properties/NI.InputThreshold33V", "Item Indent"=3, "Child Only?"=FALSE, "Glyph Index"=9}, {"Left Cell String"="SLSC-12001-030EE1BC-Mod8/bank1", "Child Text"=[], "Child Tag"="Physical Channel/bank1", "Item Indent"=1, "Child Only?"=FALSE, "Glyph Index"=31}, {"Left Cell String"="Commands", "Child Text"=[], "Child Tag"="Physical Channel/bank1/Commands", "Item Indent"=2, "Child Only?"=FALSE, "Glyph Index"=35}, {"Left Cell String"="Properties", "Child Text"=[], "Child Tag"="Physical Channel/bank1/Properties", "Item Indent"=2, "Child Only?"=FALSE, "Glyph Index"=36}, {"Left Cell String"="NI.VsupSelect", "Child Text"=["[0]Vsup_Off", "Read/Write", "I32", "Enum", "NI.VsupSource", "[0]Vsup_Off;[1]Vsup_0;[2]Vsup_1;", "[0].RW.I32.bank1.NI.VsupSelect", "Voltage source selection", "Voltage source selection for this bank. Changes to this property take effect after running the NI.ChannelConfigurationUpdate command."], "Child Tag"="Physical Channel/bank1/Properties/NI.VsupSelect", "Item Indent"=3, "Child Only?"=FALSE, "Glyph Index"=9}, {"Left Cell String"="NI.RangeEnable5V", "Child Text"=["False", "Read/Write", "Bool", "", "", "", "[0].RW.Bool.bank1.NI.RangeEnable5V", "Voltage range selection", "Enable state for this bank's voltage range. When enabled, this bank uses the NI.InputThreshold5V for the input threshold. When disabled, this bank uses the NI.InputThreshold33V for the input threshold. Changes to this property take effect after running the NI.ChannelConfigurationUpdate command."], "Child Tag"="Physical Channel/bank1/Properties/NI.RangeEnable5V", "Item Indent"=3, "Child Only?"=FALSE, "Glyph Index"=9}, {"Left Cell String"="NI.InputThreshold5V", "Child Text"=["0.7", "Read/Write", "DBL", "", "", "", "[0.7].RW.DBL.bank1.NI.InputThreshold5V", "Input threshold voltage for the 5 V range", "Input threshold voltage for this bank when its NI.RangeEnable5V is true. Changes to this property take effect after running the NI.ChannelConfigurationUpdate command."], "Child Tag"="Physical Channel/bank1/Properties/NI.InputThreshold5V", "Item Indent"=3, "Child Only?"=FALSE, "Glyph Index"=9}, {"Left Cell String"="NI.InputThreshold33V", "Child Text"=["3.706", "Read/Write", "DBL", "", "", "", "[3.706].RW.DBL.bank1.NI.InputThreshold33V", "Input threshold voltage for the 33 V range", "Input threshold voltage for this bank when its NI.RangeEnable5V is false. Changes to this property take effect after running the NI.ChannelConfigurationUpdate command."], "Child Tag"="Physical Channel/bank1/Properties/NI.InputThreshold33V", "Item Indent"=3, "Child Only?"=FALSE, "Glyph Index"=9}, {"Left Cell String"="SLSC-12001-030EE1BC-Mod8/port0/line0", "Child Text"=[], "Child Tag"="Physical Channel/port0/line0", "Item Indent"=1, "Child Only?"=FALSE, "Glyph Index"=31}, {"Left Cell String"="Commands", "Child Text"=[], "Child Tag"="Physical Channel/port0/line0/Commands", "Item Indent"=2, "Child Only?"=FALSE, "Glyph Index"=35}, {"Left Cell String"="Properties", "Child Text"=[], "Child Tag"="Physical Channel/port0/line0/Properties", "Item Indent"=2, "Child Only?"=FALSE, "Glyph Index"=36}, {"Left Cell String"="NI.Line.Index", "Child Text"=["0", "Read Only", "U32", "", "", "", "[0].R.U32.port0/line0.NI.Line.Index", "Overall index of this DIO line in the module", "This is the index of this DIO line for the aggregate module properties: NI.FrontInputBufferState, NI.RearInputBufferState, and NI.TestModeValue."], "Child Tag"="Physical Channel/port0/line0/Properties/NI.Line.Index", "Item Indent"=3, "Child Only?"=FALSE, "Glyph Index"=8}, {"Left Cell String"="NI.Line.Direction", "Child Text"=["[0]Input", "Read/Write", "I32", "Enum", "NI.Line.Direction", "[0]Input;[1]Output_Source;[2]Output_Sink;[3]Output_PushPull;", "[0].RW.I32.port0/line0.NI.Line.Direction", "DIO line direction", "Line signal flow direction through the module, relative to the front I/O connector. This property is only used when the NI.ChannelEnable for this line is set to true. Changes to this property take effect after running the NI.ChannelConfigurationUpdate command."], "Child Tag"="Physical Channel/port0/line0/Properties/NI.Line.Direction", "Item Indent"=3, "Child Only?"=FALSE, "Glyph Index"=9}, {"Left Cell String"="NI.Line.Enable", "Child Text"=["False", "Read/Write", "Bool", "", "", "", "[0].RW.Bool.port0/line0.NI.Line.Enable", "DIO line output enable", "DIO output enable for one line. When a line is enabled, the input and output buffers for the front I/O connector and the rear I/O connector of the line are configured based on the NI.Line.Direction property. When a line is not enabled, the buffers for both the front I/O connector and the rear I/O connector are configured as inputs. Changes to this property take effect after running the NI.ChannelConfigurationUpdate command."], "Child Tag"="Physical Channel/port0/line0/Properties/NI.Line.Enable", "Item Indent"=3, "Child Only?"=FALSE, "Glyph Index"=9}, {"Left Cell String"="SLSC-12001-030EE1BC-Mod8/port0/line1", "Child Text"=[], "Child Tag"="Physical Channel/port0/line1", "Item Indent"=1, "Child Only?"=FALSE, "Glyph Index"=31}, {"Left Cell String"="Commands", "Child Text"=[], "Child Tag"="Physical Channel/port0/line1/Commands", "Item Indent"=2, "Child Only?"=FALSE, "Glyph Index"=35}, {"Left Cell String"="Properties", "Child Text"=[], "Child Tag"="Physical Channel/port0/line1/Properties", "Item Indent"=2, "Child Only?"=FALSE, "Glyph Index"=36}, {"Left Cell String"="NI.Line.Index", "Child Text"=["1", "Read Only", "U32", "", "", "", "[1].R.U32.port0/line1.NI.Line.Index", "Overall index of this DIO line in the module", "This is the index of this DIO line for the aggregate module properties: NI.FrontInputBufferState, NI.RearInputBufferState, and NI.TestModeValue."], "Child Tag"="Physical Channel/port0/line1/Properties/NI.Line.Index", "Item Indent"=3, "Child Only?"=FALSE, "Glyph Index"=8}, {"Left Cell String"="NI.Line.Direction", "Child Text"=["[0]Input", "Read/Write", "I32", "Enum", "NI.Line.Direction", "[0]Input;[1]Output_Source;[2]Output_Sink;[3]Output_PushPull;", "[0].RW.I32.port0/line1.NI.Line.Direction", "DIO line direction", "Line signal flow direction through the module, relative to the front I/O connector. This property is only used when the NI.ChannelEnable for this line is set to true. Changes to this property take effect after running the NI.ChannelConfigurationUpdate command."], "Child Tag"="Physical Channel/port0/line1/Properties/NI.Line.Direction", "Item Indent"=3, "Child Only?"=FALSE, "Glyph Index"=9}, {"Left Cell String"="NI.Line.Enable", "Child Text"=["False", "Read/Write", "Bool", "", "", "", "[0].RW.Bool.port0/line1.NI.Line.Enable", "DIO line output enable", "DIO output enable for one line. When a line is enabled, the input and output buffers for the front I/O connector and the rear I/O connector of the line are configured based on the NI.Line.Direction property. When a line is not enabled, the buffers for both the front I/O connector and the rear I/O connector are configured as inputs. Changes to this property take effect after running the NI.ChannelConfigurationUpdate command."], "Child Tag"="Physical Channel/port0/line1/Properties/NI.Line.Enable", "Item Indent"=3, "Child Only?"=FALSE, "Glyph Index"=9}, {"Left Cell String"="SLSC-12001-030EE1BC-Mod8/port0/line2", "Child Text"=[], "Child Tag"="Physical Channel/port0/line2", "Item Indent"=1, "Child Only?"=FALSE, "Glyph Index"=31}, {"Left Cell String"="Commands", "Child Text"=[], "Child Tag"="Physical Channel/port0/line2/Commands", "Item Indent"=2, "Child Only?"=FALSE, "Glyph Index"=35}, {"Left Cell String"="Properties", "Child Text"=[], "Child Tag"="Physical Channel/port0/line2/Properties", "Item Indent"=2, "Child Only?"=FALSE, "Glyph Index"=36}, {"Left Cell String"="NI.Line.Index", "Child Text"=["2", "Read Only", "U32", "", "", "", "[2].R.U32.port0/line2.NI.Line.Index", "Overall index of this DIO line in the module", "This is the index of this DIO line for the aggregate module properties: NI.FrontInputBufferState, NI.RearInputBufferState, and NI.TestModeValue."], "Child Tag"="Physical Channel/port0/line2/Properties/NI.Line.Index", "Item Indent"=3, "Child Only?"=FALSE, "Glyph Index"=8}, {"Left Cell String"="NI.Line.Direction", "Child Text"=["[0]Input", "Read/Write", "I32", "Enum", "NI.Line.Direction", "[0]Input;[1]Output_Source;[2]Output_Sink;[3]Output_PushPull;", "[0].RW.I32.port0/line2.NI.Line.Direction", "DIO line direction", "Line signal flow direction through the module, relative to the front I/O connector. This property is only used when the NI.ChannelEnable for this line is set to true. Changes to this property take effect after running the NI.ChannelConfigurationUpdate command."], "Child Tag"="Physical Channel/port0/line2/Properties/NI.Line.Direction", "Item Indent"=3, "Child Only?"=FALSE, "Glyph Index"=9}, {"Left Cell String"="NI.Line.Enable", "Child Text"=["False", "Read/Write", "Bool", "", "", "", "[0].RW.Bool.port0/line2.NI.Line.Enable", "DIO line output enable", "DIO output enable for one line. When a line is enabled, the input and output buffers for the front I/O connector and the rear I/O connector of the line are configured based on the NI.Line.Direction property. When a line is not enabled, the buffers for both the front I/O connector and the rear I/O connector are configured as inputs. Changes to this property take effect after running the NI.ChannelConfigurationUpdate command."], "Child Tag"="Physical Channel/port0/line2/Properties/NI.Line.Enable", "Item Indent"=3, "Child Only?"=FALSE, "Glyph Index"=9}, {"Left Cell String"="SLSC-12001-030EE1BC-Mod8/port0/line3", "Child Text"=[], "Child Tag"="Physical Channel/port0/line3", "Item Indent"=1, "Child Only?"=FALSE, "Glyph Index"=31}, {"Left Cell String"="Commands", "Child Text"=[], "Child Tag"="Physical Channel/port0/line3/Commands", "Item Indent"=2, "Child Only?"=FALSE, "Glyph Index"=35}, {"Left Cell String"="Properties", "Child Text"=[], "Child Tag"="Physical Channel/port0/line3/Properties", "Item Indent"=2, "Child Only?"=FALSE, "Glyph Index"=36}, {"Left Cell String"="NI.Line.Index", "Child Text"=["3", "Read Only", "U32", "", "", "", "[3].R.U32.port0/line3.NI.Line.Index", "Overall index of this DIO line in the module", "This is the index of this DIO line for the aggregate module properties: NI.FrontInputBufferState, NI.RearInputBufferState, and NI.TestModeValue."], "Child Tag"="Physical Channel/port0/line3/Properties/NI.Line.Index", "Item Indent"=3, "Child Only?"=FALSE, "Glyph Index"=8}, {"Left Cell String"="NI.Line.Direction", "Child Text"=["[0]Input", "Read/Write", "I32", "Enum", "NI.Line.Direction", "[0]Input;[1]Output_Source;[2]Output_Sink;[3]Output_PushPull;", "[0].RW.I32.port0/line3.NI.Line.Direction", "DIO line direction", "Line signal flow direction through the module, relative to the front I/O connector. This property is only used when the NI.ChannelEnable for this line is set to true. Changes to this property take effect after running the NI.ChannelConfigurationUpdate command."], "Child Tag"="Physical Channel/port0/line3/Properties/NI.Line.Direction", "Item Indent"=3, "Child Only?"=FALSE, "Glyph Index"=9}, {"Left Cell String"="NI.Line.Enable", "Child Text"=["False", "Read/Write", "Bool", "", "", "", "[0].RW.Bool.port0/line3.NI.Line.Enable", "DIO line output enable", "DIO output enable for one line. When a line is enabled, the input and output buffers for the front I/O connector and the rear I/O connector of the line are configured based on the NI.Line.Direction property. When a line is not enabled, the buffers for both the front I/O connector and the rear I/O connector are configured as inputs. Changes to this property take effect after running the NI.ChannelConfigurationUpdate command."], "Child Tag"="Physical Channel/port0/line3/Properties/NI.Line.Enable", "Item Indent"=3, "Child Only?"=FALSE, "Glyph Index"=9}, {"Left Cell String"="SLSC-12001-030EE1BC-Mod8/port0/line4", "Child Text"=[], "Child Tag"="Physical Channel/port0/line4", "Item Indent"=1, "Child Only?"=FALSE, "Glyph Index"=31}, {"Left Cell String"="Commands", "Child Text"=[], "Child Tag"="Physical Channel/port0/line4/Commands", "Item Indent"=2, "Child Only?"=FALSE, "Glyph Index"=35}, {"Left Cell String"="Properties", "Child Text"=[], "Child Tag"="Physical Channel/port0/line4/Properties", "Item Indent"=2, "Child Only?"=FALSE, "Glyph Index"=36}, {"Left Cell String"="NI.Line.Index", "Child Text"=["4", "Read Only", "U32", "", "", "", "[4].R.U32.port0/line4.NI.Line.Index", "Overall index of this DIO line in the module", "This is the index of this DIO line for the aggregate module properties: NI.FrontInputBufferState, NI.RearInputBufferState, and NI.TestModeValue."], "Child Tag"="Physical Channel/port0/line4/Properties/NI.Line.Index", "Item Indent"=3, "Child Only?"=FALSE, "Glyph Index"=8}, {"Left Cell String"="NI.Line.Direction", "Child Text"=["[0]Input", "Read/Write", "I32", "Enum", "NI.Line.Direction", "[0]Input;[1]Output_Source;[2]Output_Sink;[3]Output_PushPull;", "[0].RW.I32.port0/line4.NI.Line.Direction", "DIO line direction", "Line signal flow direction through the module, relative to the front I/O connector. This property is only used when the NI.ChannelEnable for this line is set to true. Changes to this property take effect after running the NI.ChannelConfigurationUpdate command."], "Child Tag"="Physical Channel/port0/line4/Properties/NI.Line.Direction", "Item Indent"=3, "Child Only?"=FALSE, "Glyph Index"=9}, {"Left Cell String"="NI.Line.Enable", "Child Text"=["False", "Read/Write", "Bool", "", "", "", "[0].RW.Bool.port0/line4.NI.Line.Enable", "DIO line output enable", "DIO output enable for one line. When a line is enabled, the input and output buffers for the front I/O connector and the rear I/O connector of the line are configured based on the NI.Line.Direction property. When a line is not enabled, the buffers for both the front I/O connector and the rear I/O connector are configured as inputs. Changes to this property take effect after running the NI.ChannelConfigurationUpdate command."], "Child Tag"="Physical Channel/port0/line4/Properties/NI.Line.Enable", "Item Indent"=3, "Child Only?"=FALSE, "Glyph Index"=9}, {"Left Cell String"="SLSC-12001-030EE1BC-Mod8/port0/line5", "Child Text"=[], "Child Tag"="Physical Channel/port0/line5", "Item Indent"=1, "Child Only?"=FALSE, "Glyph Index"=31}, {"Left Cell String"="Commands", "Child Text"=[], "Child Tag"="Physical Channel/port0/line5/Commands", "Item Indent"=2, "Child Only?"=FALSE, "Glyph Index"=35}, {"Left Cell String"="Properties", "Child Text"=[], "Child Tag"="Physical Channel/port0/line5/Properties", "Item Indent"=2, "Child Only?"=FALSE, "Glyph Index"=36}, {"Left Cell String"="NI.Line.Index", "Child Text"=["5", "Read Only", "U32", "", "", "", "[5].R.U32.port0/line5.NI.Line.Index", "Overall index of this DIO line in the module", "This is the index of this DIO line for the aggregate module properties: NI.FrontInputBufferState, NI.RearInputBufferState, and NI.TestModeValue."], "Child Tag"="Physical Channel/port0/line5/Properties/NI.Line.Index", "Item Indent"=3, "Child Only?"=FALSE, "Glyph Index"=8}, {"Left Cell String"="NI.Line.Direction", "Child Text"=["[0]Input", "Read/Write", "I32", "Enum", "NI.Line.Direction", "[0]Input;[1]Output_Source;[2]Output_Sink;[3]Output_PushPull;", "[0].RW.I32.port0/line5.NI.Line.Direction", "DIO line direction", "Line signal flow direction through the module, relative to the front I/O connector. This property is only used when the NI.ChannelEnable for this line is set to true. Changes to this property take effect after running the NI.ChannelConfigurationUpdate command."], "Child Tag"="Physical Channel/port0/line5/Properties/NI.Line.Direction", "Item Indent"=3, "Child Only?"=FALSE, "Glyph Index"=9}, {"Left Cell String"="NI.Line.Enable", "Child Text"=["False", "Read/Write", "Bool", "", "", "", "[0].RW.Bool.port0/line5.NI.Line.Enable", "DIO line output enable", "DIO output enable for one line. When a line is enabled, the input and output buffers for the front I/O connector and the rear I/O connector of the line are configured based on the NI.Line.Direction property. When a line is not enabled, the buffers for both the front I/O connector and the rear I/O connector are configured as inputs. Changes to this property take effect after running the NI.ChannelConfigurationUpdate command."], "Child Tag"="Physical Channel/port0/line5/Properties/NI.Line.Enable", "Item Indent"=3, "Child Only?"=FALSE, "Glyph Index"=9}, {"Left Cell String"="SLSC-12001-030EE1BC-Mod8/port0/line6", "Child Text"=[], "Child Tag"="Physical Channel/port0/line6", "Item Indent"=1, "Child Only?"=FALSE, "Glyph Index"=31}, {"Left Cell String"="Commands", "Child Text"=[], "Child Tag"="Physical Channel/port0/line6/Commands", "Item Indent"=2, "Child Only?"=FALSE, "Glyph Index"=35}, {"Left Cell String"="Properties", "Child Text"=[], "Child Tag"="Physical Channel/port0/line6/Properties", "Item Indent"=2, "Child Only?"=FALSE, "Glyph Index"=36}, {"Left Cell String"="NI.Line.Index", "Child Text"=["6", "Read Only", "U32", "", "", "", "[6].R.U32.port0/line6.NI.Line.Index", "Overall index of this DIO line in the module", "This is the index of this DIO line for the aggregate module properties: NI.FrontInputBufferState, NI.RearInputBufferState, and NI.TestModeValue."], "Child Tag"="Physical Channel/port0/line6/Properties/NI.Line.Index", "Item Indent"=3, "Child Only?"=FALSE, "Glyph Index"=8}, {"Left Cell String"="NI.Line.Direction", "Child Text"=["[0]Input", "Read/Write", "I32", "Enum", "NI.Line.Direction", "[0]Input;[1]Output_Source;[2]Output_Sink;[3]Output_PushPull;", "[0].RW.I32.port0/line6.NI.Line.Direction", "DIO line direction", "Line signal flow direction through the module, relative to the front I/O connector. This property is only used when the NI.ChannelEnable for this line is set to true. Changes to this property take effect after running the NI.ChannelConfigurationUpdate command."], "Child Tag"="Physical Channel/port0/line6/Properties/NI.Line.Direction", "Item Indent"=3, "Child Only?"=FALSE, "Glyph Index"=9}, {"Left Cell String"="NI.Line.Enable", "Child Text"=["False", "Read/Write", "Bool", "", "", "", "[0].RW.Bool.port0/line6.NI.Line.Enable", "DIO line output enable", "DIO output enable for one line. When a line is enabled, the input and output buffers for the front I/O connector and the rear I/O connector of the line are configured based on the NI.Line.Direction property. When a line is not enabled, the buffers for both the front I/O connector and the rear I/O connector are configured as inputs. Changes to this property take effect after running the NI.ChannelConfigurationUpdate command."], "Child Tag"="Physical Channel/port0/line6/Properties/NI.Line.Enable", "Item Indent"=3, "Child Only?"=FALSE, "Glyph Index"=9}, {"Left Cell String"="SLSC-12001-030EE1BC-Mod8/port0/line7", "Child Text"=[], "Child Tag"="Physical Channel/port0/line7", "Item Indent"=1, "Child Only?"=FALSE, "Glyph Index"=31}, {"Left Cell String"="Commands", "Child Text"=[], "Child Tag"="Physical Channel/port0/line7/Commands", "Item Indent"=2, "Child Only?"=FALSE, "Glyph Index"=35}, {"Left Cell String"="Properties", "Child Text"=[], "Child Tag"="Physical Channel/port0/line7/Properties", "Item Indent"=2, "Child Only?"=FALSE, "Glyph Index"=36}, {"Left Cell String"="NI.Line.Index", "Child Text"=["7", "Read Only", "U32", "", "", "", "[7].R.U32.port0/line7.NI.Line.Index", "Overall index of this DIO line in the module", "This is the index of this DIO line for the aggregate module properties: NI.FrontInputBufferState, NI.RearInputBufferState, and NI.TestModeValue."], "Child Tag"="Physical Channel/port0/line7/Properties/NI.Line.Index", "Item Indent"=3, "Child Only?"=FALSE, "Glyph Index"=8}, {"Left Cell String"="NI.Line.Direction", "Child Text"=["[0]Input", "Read/Write", "I32", "Enum", "NI.Line.Direction", "[0]Input;[1]Output_Source;[2]Output_Sink;[3]Output_PushPull;", "[0].RW.I32.port0/line7.NI.Line.Direction", "DIO line direction", "Line signal flow direction through the module, relative to the front I/O connector. This property is only used when the NI.ChannelEnable for this line is set to true. Changes to this property take effect after running the NI.ChannelConfigurationUpdate command."], "Child Tag"="Physical Channel/port0/line7/Properties/NI.Line.Direction", "Item Indent"=3, "Child Only?"=FALSE, "Glyph Index"=9}, {"Left Cell String"="NI.Line.Enable", "Child Text"=["False", "Read/Write", "Bool", "", "", "", "[0].RW.Bool.port0/line7.NI.Line.Enable", "DIO line output enable", "DIO output enable for one line. When a line is enabled, the input and output buffers for the front I/O connector and the rear I/O connector of the line are configured based on the NI.Line.Direction property. When a line is not enabled, the buffers for both the front I/O connector and the rear I/O connector are configured as inputs. Changes to this property take effect after running the NI.ChannelConfigurationUpdate command."], "Child Tag"="Physical Channel/port0/line7/Properties/NI.Line.Enable", "Item Indent"=3, "Child Only?"=FALSE, "Glyph Index"=9}, {"Left Cell String"="SLSC-12001-030EE1BC-Mod8/port1/line0", "Child Text"=[], "Child Tag"="Physical Channel/port1/line0", "Item Indent"=1, "Child Only?"=FALSE, "Glyph Index"=31}, {"Left Cell String"="Commands", "Child Text"=[], "Child Tag"="Physical Channel/port1/line0/Commands", "Item Indent"=2, "Child Only?"=FALSE, "Glyph Index"=35}, {"Left Cell String"="Properties", "Child Text"=[], "Child Tag"="Physical Channel/port1/line0/Properties", "Item Indent"=2, "Child Only?"=FALSE, "Glyph Index"=36}, {"Left Cell String"="NI.Line.Index", "Child Text"=["8", "Read Only", "U32", "", "", "", "[8].R.U32.port1/line0.NI.Line.Index", "Overall index of this DIO line in the module", "This is the index of this DIO line for the aggregate module properties: NI.FrontInputBufferState, NI.RearInputBufferState, and NI.TestModeValue."], "Child Tag"="Physical Channel/port1/line0/Properties/NI.Line.Index", "Item Indent"=3, "Child Only?"=FALSE, "Glyph Index"=8}, {"Left Cell String"="NI.Line.Direction", "Child Text"=["[0]Input", "Read/Write", "I32", "Enum", "NI.Line.Direction", "[0]Input;[1]Output_Source;[2]Output_Sink;[3]Output_PushPull;", "[0].RW.I32.port1/line0.NI.Line.Direction", "DIO line direction", "Line signal flow direction through the module, relative to the front I/O connector. This property is only used when the NI.ChannelEnable for this line is set to true. Changes to this property take effect after running the NI.ChannelConfigurationUpdate command."], "Child Tag"="Physical Channel/port1/line0/Properties/NI.Line.Direction", "Item Indent"=3, "Child Only?"=FALSE, "Glyph Index"=9}, {"Left Cell String"="NI.Line.Enable", "Child Text"=["False", "Read/Write", "Bool", "", "", "", "[0].RW.Bool.port1/line0.NI.Line.Enable", "DIO line output enable", "DIO output enable for one line. When a line is enabled, the input and output buffers for the front I/O connector and the rear I/O connector of the line are configured based on the NI.Line.Direction property. When a line is not enabled, the buffers for both the front I/O connector and the rear I/O connector are configured as inputs. Changes to this property take effect after running the NI.ChannelConfigurationUpdate command."], "Child Tag"="Physical Channel/port1/line0/Properties/NI.Line.Enable", "Item Indent"=3, "Child Only?"=FALSE, "Glyph Index"=9}, {"Left Cell String"="SLSC-12001-030EE1BC-Mod8/port1/line1", "Child Text"=[], "Child Tag"="Physical Channel/port1/line1", "Item Indent"=1, "Child Only?"=FALSE, "Glyph Index"=31}, {"Left Cell String"="Commands", "Child Text"=[], "Child Tag"="Physical Channel/port1/line1/Commands", "Item Indent"=2, "Child Only?"=FALSE, "Glyph Index"=35}, {"Left Cell String"="Properties", "Child Text"=[], "Child Tag"="Physical Channel/port1/line1/Properties", "Item Indent"=2, "Child Only?"=FALSE, "Glyph Index"=36}, {"Left Cell String"="NI.Line.Index", "Child Text"=["9", "Read Only", "U32", "", "", "", "[9].R.U32.port1/line1.NI.Line.Index", "Overall index of this DIO line in the module", "This is the index of this DIO line for the aggregate module properties: NI.FrontInputBufferState, NI.RearInputBufferState, and NI.TestModeValue."], "Child Tag"="Physical Channel/port1/line1/Properties/NI.Line.Index", "Item Indent"=3, "Child Only?"=FALSE, "Glyph Index"=8}, {"Left Cell String"="NI.Line.Direction", "Child Text"=["[0]Input", "Read/Write", "I32", "Enum", "NI.Line.Direction", "[0]Input;[1]Output_Source;[2]Output_Sink;[3]Output_PushPull;", "[0].RW.I32.port1/line1.NI.Line.Direction", "DIO line direction", "Line signal flow direction through the module, relative to the front I/O connector. This property is only used when the NI.ChannelEnable for this line is set to true. Changes to this property take effect after running the NI.ChannelConfigurationUpdate command."], "Child Tag"="Physical Channel/port1/line1/Properties/NI.Line.Direction", "Item Indent"=3, "Child Only?"=FALSE, "Glyph Index"=9}, {"Left Cell String"="NI.Line.Enable", "Child Text"=["False", "Read/Write", "Bool", "", "", "", "[0].RW.Bool.port1/line1.NI.Line.Enable", "DIO line output enable", "DIO output enable for one line. When a line is enabled, the input and output buffers for the front I/O connector and the rear I/O connector of the line are configured based on the NI.Line.Direction property. When a line is not enabled, the buffers for both the front I/O connector and the rear I/O connector are configured as inputs. Changes to this property take effect after running the NI.ChannelConfigurationUpdate command."], "Child Tag"="Physical Channel/port1/line1/Properties/NI.Line.Enable", "Item Indent"=3, "Child Only?"=FALSE, "Glyph Index"=9}, {"Left Cell String"="SLSC-12001-030EE1BC-Mod8/port1/line2", "Child Text"=[], "Child Tag"="Physical Channel/port1/line2", "Item Indent"=1, "Child Only?"=FALSE, "Glyph Index"=31}, {"Left Cell String"="Commands", "Child Text"=[], "Child Tag"="Physical Channel/port1/line2/Commands", "Item Indent"=2, "Child Only?"=FALSE, "Glyph Index"=35}, {"Left Cell String"="Properties", "Child Text"=[], "Child Tag"="Physical Channel/port1/line2/Properties", "Item Indent"=2, "Child Only?"=FALSE, "Glyph Index"=36}, {"Left Cell String"="NI.Line.Index", "Child Text"=["A", "Read Only", "U32", "", "", "", "[10].R.U32.port1/line2.NI.Line.Index", "Overall index of this DIO line in the module", "This is the index of this DIO line for the aggregate module properties: NI.FrontInputBufferState, NI.RearInputBufferState, and NI.TestModeValue."], "Child Tag"="Physical Channel/port1/line2/Properties/NI.Line.Index", "Item Indent"=3, "Child Only?"=FALSE, "Glyph Index"=8}, {"Left Cell String"="NI.Line.Direction", "Child Text"=["[0]Input", "Read/Write", "I32", "Enum", "NI.Line.Direction", "[0]Input;[1]Output_Source;[2]Output_Sink;[3]Output_PushPull;", "[0].RW.I32.port1/line2.NI.Line.Direction", "DIO line direction", "Line signal flow direction through the module, relative to the front I/O connector. This property is only used when the NI.ChannelEnable for this line is set to true. Changes to this property take effect after running the NI.ChannelConfigurationUpdate command."], "Child Tag"="Physical Channel/port1/line2/Properties/NI.Line.Direction", "Item Indent"=3, "Child Only?"=FALSE, "Glyph Index"=9}, {"Left Cell String"="NI.Line.Enable", "Child Text"=["False", "Read/Write", "Bool", "", "", "", "[0].RW.Bool.port1/line2.NI.Line.Enable", "DIO line output enable", "DIO output enable for one line. When a line is enabled, the input and output buffers for the front I/O connector and the rear I/O connector of the line are configured based on the NI.Line.Direction property. When a line is not enabled, the buffers for both the front I/O connector and the rear I/O connector are configured as inputs. Changes to this property take effect after running the NI.ChannelConfigurationUpdate command."], "Child Tag"="Physical Channel/port1/line2/Properties/NI.Line.Enable", "Item Indent"=3, "Child Only?"=FALSE, "Glyph Index"=9}, {"Left Cell String"="SLSC-12001-030EE1BC-Mod8/port1/line3", "Child Text"=[], "Child Tag"="Physical Channel/port1/line3", "Item Indent"=1, "Child Only?"=FALSE, "Glyph Index"=31}, {"Left Cell String"="Commands", "Child Text"=[], "Child Tag"="Physical Channel/port1/line3/Commands", "Item Indent"=2, "Child Only?"=FALSE, "Glyph Index"=35}, {"Left Cell String"="Properties", "Child Text"=[], "Child Tag"="Physical Channel/port1/line3/Properties", "Item Indent"=2, "Child Only?"=FALSE, "Glyph Index"=36}, {"Left Cell String"="NI.Line.Index", "Child Text"=["B", "Read Only", "U32", "", "", "", "[11].R.U32.port1/line3.NI.Line.Index", "Overall index of this DIO line in the module", "This is the index of this DIO line for the aggregate module properties: NI.FrontInputBufferState, NI.RearInputBufferState, and NI.TestModeValue."], "Child Tag"="Physical Channel/port1/line3/Properties/NI.Line.Index", "Item Indent"=3, "Child Only?"=FALSE, "Glyph Index"=8}, {"Left Cell String"="NI.Line.Direction", "Child Text"=["[0]Input", "Read/Write", "I32", "Enum", "NI.Line.Direction", "[0]Input;[1]Output_Source;[2]Output_Sink;[3]Output_PushPull;", "[0].RW.I32.port1/line3.NI.Line.Direction", "DIO line direction", "Line signal flow direction through the module, relative to the front I/O connector. This property is only used when the NI.ChannelEnable for this line is set to true. Changes to this property take effect after running the NI.ChannelConfigurationUpdate command."], "Child Tag"="Physical Channel/port1/line3/Properties/NI.Line.Direction", "Item Indent"=3, "Child Only?"=FALSE, "Glyph Index"=9}, {"Left Cell String"="NI.Line.Enable", "Child Text"=["False", "Read/Write", "Bool", "", "", "", "[0].RW.Bool.port1/line3.NI.Line.Enable", "DIO line output enable", "DIO output enable for one line. When a line is enabled, the input and output buffers for the front I/O connector and the rear I/O connector of the line are configured based on the NI.Line.Direction property. When a line is not enabled, the buffers for both the front I/O connector and the rear I/O connector are configured as inputs. Changes to this property take effect after running the NI.ChannelConfigurationUpdate command."], "Child Tag"="Physical Channel/port1/line3/Properties/NI.Line.Enable", "Item Indent"=3, "Child Only?"=FALSE, "Glyph Index"=9}, {"Left Cell String"="SLSC-12001-030EE1BC-Mod8/port1/line4", "Child Text"=[], "Child Tag"="Physical Channel/port1/line4", "Item Indent"=1, "Child Only?"=FALSE, "Glyph Index"=31}, {"Left Cell String"="Commands", "Child Text"=[], "Child Tag"="Physical Channel/port1/line4/Commands", "Item Indent"=2, "Child Only?"=FALSE, "Glyph Index"=35}, {"Left Cell String"="Properties", "Child Text"=[], "Child Tag"="Physical Channel/port1/line4/Properties", "Item Indent"=2, "Child Only?"=FALSE, "Glyph Index"=36}, {"Left Cell String"="NI.Line.Index", "Child Text"=["C", "Read Only", "U32", "", "", "", "[12].R.U32.port1/line4.NI.Line.Index", "Overall index of this DIO line in the module", "This is the index of this DIO line for the aggregate module properties: NI.FrontInputBufferState, NI.RearInputBufferState, and NI.TestModeValue."], "Child Tag"="Physical Channel/port1/line4/Properties/NI.Line.Index", "Item Indent"=3, "Child Only?"=FALSE, "Glyph Index"=8}, {"Left Cell String"="NI.Line.Direction", "Child Text"=["[0]Input", "Read/Write", "I32", "Enum", "NI.Line.Direction", "[0]Input;[1]Output_Source;[2]Output_Sink;[3]Output_PushPull;", "[0].RW.I32.port1/line4.NI.Line.Direction", "DIO line direction", "Line signal flow direction through the module, relative to the front I/O connector. This property is only used when the NI.ChannelEnable for this line is set to true. Changes to this property take effect after running the NI.ChannelConfigurationUpdate command."], "Child Tag"="Physical Channel/port1/line4/Properties/NI.Line.Direction", "Item Indent"=3, "Child Only?"=FALSE, "Glyph Index"=9}, {"Left Cell String"="NI.Line.Enable", "Child Text"=["False", "Read/Write", "Bool", "", "", "", "[0].RW.Bool.port1/line4.NI.Line.Enable", "DIO line output enable", "DIO output enable for one line. When a line is enabled, the input and output buffers for the front I/O connector and the rear I/O connector of the line are configured based on the NI.Line.Direction property. When a line is not enabled, the buffers for both the front I/O connector and the rear I/O connector are configured as inputs. Changes to this property take effect after running the NI.ChannelConfigurationUpdate command."], "Child Tag"="Physical Channel/port1/line4/Properties/NI.Line.Enable", "Item Indent"=3, "Child Only?"=FALSE, "Glyph Index"=9}, {"Left Cell String"="SLSC-12001-030EE1BC-Mod8/port1/line5", "Child Text"=[], "Child Tag"="Physical Channel/port1/line5", "Item Indent"=1, "Child Only?"=FALSE, "Glyph Index"=31}, {"Left Cell String"="Commands", "Child Text"=[], "Child Tag"="Physical Channel/port1/line5/Commands", "Item Indent"=2, "Child Only?"=FALSE, "Glyph Index"=35}, {"Left Cell String"="Properties", "Child Text"=[], "Child Tag"="Physical Channel/port1/line5/Properties", "Item Indent"=2, "Child Only?"=FALSE, "Glyph Index"=36}, {"Left Cell String"="NI.Line.Index", "Child Text"=["D", "Read Only", "U32", "", "", "", "[13].R.U32.port1/line5.NI.Line.Index", "Overall index of this DIO line in the module", "This is the index of this DIO line for the aggregate module properties: NI.FrontInputBufferState, NI.RearInputBufferState, and NI.TestModeValue."], "Child Tag"="Physical Channel/port1/line5/Properties/NI.Line.Index", "Item Indent"=3, "Child Only?"=FALSE, "Glyph Index"=8}, {"Left Cell String"="NI.Line.Direction", "Child Text"=["[0]Input", "Read/Write", "I32", "Enum", "NI.Line.Direction", "[0]Input;[1]Output_Source;[2]Output_Sink;[3]Output_PushPull;", "[0].RW.I32.port1/line5.NI.Line.Direction", "DIO line direction", "Line signal flow direction through the module, relative to the front I/O connector. This property is only used when the NI.ChannelEnable for this line is set to true. Changes to this property take effect after running the NI.ChannelConfigurationUpdate command."], "Child Tag"="Physical Channel/port1/line5/Properties/NI.Line.Direction", "Item Indent"=3, "Child Only?"=FALSE, "Glyph Index"=9}, {"Left Cell String"="NI.Line.Enable", "Child Text"=["False", "Read/Write", "Bool", "", "", "", "[0].RW.Bool.port1/line5.NI.Line.Enable", "DIO line output enable", "DIO output enable for one line. When a line is enabled, the input and output buffers for the front I/O connector and the rear I/O connector of the line are configured based on the NI.Line.Direction property. When a line is not enabled, the buffers for both the front I/O connector and the rear I/O connector are configured as inputs. Changes to this property take effect after running the NI.ChannelConfigurationUpdate command."], "Child Tag"="Physical Channel/port1/line5/Properties/NI.Line.Enable", "Item Indent"=3, "Child Only?"=FALSE, "Glyph Index"=9}, {"Left Cell String"="SLSC-12001-030EE1BC-Mod8/port1/line6", "Child Text"=[], "Child Tag"="Physical Channel/port1/line6", "Item Indent"=1, "Child Only?"=FALSE, "Glyph Index"=31}, {"Left Cell String"="Commands", "Child Text"=[], "Child Tag"="Physical Channel/port1/line6/Commands", "Item Indent"=2, "Child Only?"=FALSE, "Glyph Index"=35}, {"Left Cell String"="Properties", "Child Text"=[], "Child Tag"="Physical Channel/port1/line6/Properties", "Item Indent"=2, "Child Only?"=FALSE, "Glyph Index"=36}, {"Left Cell String"="NI.Line.Index", "Child Text"=["E", "Read Only", "U32", "", "", "", "[14].R.U32.port1/line6.NI.Line.Index", "Overall index of this DIO line in the module", "This is the index of this DIO line for the aggregate module properties: NI.FrontInputBufferState, NI.RearInputBufferState, and NI.TestModeValue."], "Child Tag"="Physical Channel/port1/line6/Properties/NI.Line.Index", "Item Indent"=3, "Child Only?"=FALSE, "Glyph Index"=8}, {"Left Cell String"="NI.Line.Direction", "Child Text"=["[0]Input", "Read/Write", "I32", "Enum", "NI.Line.Direction", "[0]Input;[1]Output_Source;[2]Output_Sink;[3]Output_PushPull;", "[0].RW.I32.port1/line6.NI.Line.Direction", "DIO line direction", "Line signal flow direction through the module, relative to the front I/O connector. This property is only used when the NI.ChannelEnable for this line is set to true. Changes to this property take effect after running the NI.ChannelConfigurationUpdate command."], "Child Tag"="Physical Channel/port1/line6/Properties/NI.Line.Direction", "Item Indent"=3, "Child Only?"=FALSE, "Glyph Index"=9}, {"Left Cell String"="NI.Line.Enable", "Child Text"=["False", "Read/Write", "Bool", "", "", "", "[0].RW.Bool.port1/line6.NI.Line.Enable", "DIO line output enable", "DIO output enable for one line. When a line is enabled, the input and output buffers for the front I/O connector and the rear I/O connector of the line are configured based on the NI.Line.Direction property. When a line is not enabled, the buffers for both the front I/O connector and the rear I/O connector are configured as inputs. Changes to this property take effect after running the NI.ChannelConfigurationUpdate command."], "Child Tag"="Physical Channel/port1/line6/Properties/NI.Line.Enable", "Item Indent"=3, "Child Only?"=FALSE, "Glyph Index"=9}, {"Left Cell String"="SLSC-12001-030EE1BC-Mod8/port1/line7", "Child Text"=[], "Child Tag"="Physical Channel/port1/line7", "Item Indent"=1, "Child Only?"=FALSE, "Glyph Index"=31}, {"Left Cell String"="Commands", "Child Text"=[], "Child Tag"="Physical Channel/port1/line7/Commands", "Item Indent"=2, "Child Only?"=FALSE, "Glyph Index"=35}, {"Left Cell String"="Properties", "Child Text"=[], "Child Tag"="Physical Channel/port1/line7/Properties", "Item Indent"=2, "Child Only?"=FALSE, "Glyph Index"=36}, {"Left Cell String"="NI.Line.Index", "Child Text"=["F", "Read Only", "U32", "", "", "", "[15].R.U32.port1/line7.NI.Line.Index", "Overall index of this DIO line in the module", "This is the index of this DIO line for the aggregate module properties: NI.FrontInputBufferState, NI.RearInputBufferState, and NI.TestModeValue."], "Child Tag"="Physical Channel/port1/line7/Properties/NI.Line.Index", "Item Indent"=3, "Child Only?"=FALSE, "Glyph Index"=8}, {"Left Cell String"="NI.Line.Direction", "Child Text"=["[0]Input", "Read/Write", "I32", "Enum", "NI.Line.Direction", "[0]Input;[1]Output_Source;[2]Output_Sink;[3]Output_PushPull;", "[0].RW.I32.port1/line7.NI.Line.Direction", "DIO line direction", "Line signal flow direction through the module, relative to the front I/O connector. This property is only used when the NI.ChannelEnable for this line is set to true. Changes to this property take effect after running the NI.ChannelConfigurationUpdate command."], "Child Tag"="Physical Channel/port1/line7/Properties/NI.Line.Direction", "Item Indent"=3, "Child Only?"=FALSE, "Glyph Index"=9}, {"Left Cell String"="NI.Line.Enable", "Child Text"=["False", "Read/Write", "Bool", "", "", "", "[0].RW.Bool.port1/line7.NI.Line.Enable", "DIO line output enable", "DIO output enable for one line. When a line is enabled, the input and output buffers for the front I/O connector and the rear I/O connector of the line are configured based on the NI.Line.Direction property. When a line is not enabled, the buffers for both the front I/O connector and the rear I/O connector are configured as inputs. Changes to this property take effect after running the NI.ChannelConfigurationUpdate command."], "Child Tag"="Physical Channel/port1/line7/Properties/NI.Line.Enable", "Item Indent"=3, "Child Only?"=FALSE, "Glyph Index"=9}, {"Left Cell String"="SLSC-12001-030EE1BC-Mod8/port2/line0", "Child Text"=[], "Child Tag"="Physical Channel/port2/line0", "Item Indent"=1, "Child Only?"=FALSE, "Glyph Index"=31}, {"Left Cell String"="Commands", "Child Text"=[], "Child Tag"="Physical Channel/port2/line0/Commands", "Item Indent"=2, "Child Only?"=FALSE, "Glyph Index"=35}, {"Left Cell String"="Properties", "Child Text"=[], "Child Tag"="Physical Channel/port2/line0/Properties", "Item Indent"=2, "Child Only?"=FALSE, "Glyph Index"=36}, {"Left Cell String"="NI.Line.Index", "Child Text"=["10", "Read Only", "U32", "", "", "", "[16].R.U32.port2/line0.NI.Line.Index", "Overall index of this DIO line in the module", "This is the index of this DIO line for the aggregate module properties: NI.FrontInputBufferState, NI.RearInputBufferState, and NI.TestModeValue."], "Child Tag"="Physical Channel/port2/line0/Properties/NI.Line.Index", "Item Indent"=3, "Child Only?"=FALSE, "Glyph Index"=8}, {"Left Cell String"="NI.Line.Direction", "Child Text"=["[0]Input", "Read/Write", "I32", "Enum", "NI.Line.Direction", "[0]Input;[1]Output_Source;[2]Output_Sink;[3]Output_PushPull;", "[0].RW.I32.port2/line0.NI.Line.Direction", "DIO line direction", "Line signal flow direction through the module, relative to the front I/O connector. This property is only used when the NI.ChannelEnable for this line is set to true. Changes to this property take effect after running the NI.ChannelConfigurationUpdate command."], "Child Tag"="Physical Channel/port2/line0/Properties/NI.Line.Direction", "Item Indent"=3, "Child Only?"=FALSE, "Glyph Index"=9}, {"Left Cell String"="NI.Line.Enable", "Child Text"=["False", "Read/Write", "Bool", "", "", "", "[0].RW.Bool.port2/line0.NI.Line.Enable", "DIO line output enable", "DIO output enable for one line. When a line is enabled, the input and output buffers for the front I/O connector and the rear I/O connector of the line are configured based on the NI.Line.Direction property. When a line is not enabled, the buffers for both the front I/O connector and the rear I/O connector are configured as inputs. Changes to this property take effect after running the NI.ChannelConfigurationUpdate command."], "Child Tag"="Physical Channel/port2/line0/Properties/NI.Line.Enable", "Item Indent"=3, "Child Only?"=FALSE, "Glyph Index"=9}, {"Left Cell String"="SLSC-12001-030EE1BC-Mod8/port2/line1", "Child Text"=[], "Child Tag"="Physical Channel/port2/line1", "Item Indent"=1, "Child Only?"=FALSE, "Glyph Index"=31}, {"Left Cell String"="Commands", "Child Text"=[], "Child Tag"="Physical Channel/port2/line1/Commands", "Item Indent"=2, "Child Only?"=FALSE, "Glyph Index"=35}, {"Left Cell String"="Properties", "Child Text"=[], "Child Tag"="Physical Channel/port2/line1/Properties", "Item Indent"=2, "Child Only?"=FALSE, "Glyph Index"=36}, {"Left Cell String"="NI.Line.Index", "Child Text"=["11", "Read Only", "U32", "", "", "", "[17].R.U32.port2/line1.NI.Line.Index", "Overall index of this DIO line in the module", "This is the index of this DIO line for the aggregate module properties: NI.FrontInputBufferState, NI.RearInputBufferState, and NI.TestModeValue."], "Child Tag"="Physical Channel/port2/line1/Properties/NI.Line.Index", "Item Indent"=3, "Child Only?"=FALSE, "Glyph Index"=8}, {"Left Cell String"="NI.Line.Direction", "Child Text"=["[0]Input", "Read/Write", "I32", "Enum", "NI.Line.Direction", "[0]Input;[1]Output_Source;[2]Output_Sink;[3]Output_PushPull;", "[0].RW.I32.port2/line1.NI.Line.Direction", "DIO line direction", "Line signal flow direction through the module, relative to the front I/O connector. This property is only used when the NI.ChannelEnable for this line is set to true. Changes to this property take effect after running the NI.ChannelConfigurationUpdate command."], "Child Tag"="Physical Channel/port2/line1/Properties/NI.Line.Direction", "Item Indent"=3, "Child Only?"=FALSE, "Glyph Index"=9}, {"Left Cell String"="NI.Line.Enable", "Child Text"=["False", "Read/Write", "Bool", "", "", "", "[0].RW.Bool.port2/line1.NI.Line.Enable", "DIO line output enable", "DIO output enable for one line. When a line is enabled, the input and output buffers for the front I/O connector and the rear I/O connector of the line are configured based on the NI.Line.Direction property. When a line is not enabled, the buffers for both the front I/O connector and the rear I/O connector are configured as inputs. Changes to this property take effect after running the NI.ChannelConfigurationUpdate command."], "Child Tag"="Physical Channel/port2/line1/Properties/NI.Line.Enable", "Item Indent"=3, "Child Only?"=FALSE, "Glyph Index"=9}, {"Left Cell String"="SLSC-12001-030EE1BC-Mod8/port2/line2", "Child Text"=[], "Child Tag"="Physical Channel/port2/line2", "Item Indent"=1, "Child Only?"=FALSE, "Glyph Index"=31}, {"Left Cell String"="Commands", "Child Text"=[], "Child Tag"="Physical Channel/port2/line2/Commands", "Item Indent"=2, "Child Only?"=FALSE, "Glyph Index"=35}, {"Left Cell String"="Properties", "Child Text"=[], "Child Tag"="Physical Channel/port2/line2/Properties", "Item Indent"=2, "Child Only?"=FALSE, "Glyph Index"=36}, {"Left Cell String"="NI.Line.Index", "Child Text"=["12", "Read Only", "U32", "", "", "", "[18].R.U32.port2/line2.NI.Line.Index", "Overall index of this DIO line in the module", "This is the index of this DIO line for the aggregate module properties: NI.FrontInputBufferState, NI.RearInputBufferState, and NI.TestModeValue."], "Child Tag"="Physical Channel/port2/line2/Properties/NI.Line.Index", "Item Indent"=3, "Child Only?"=FALSE, "Glyph Index"=8}, {"Left Cell String"="NI.Line.Direction", "Child Text"=["[0]Input", "Read/Write", "I32", "Enum", "NI.Line.Direction", "[0]Input;[1]Output_Source;[2]Output_Sink;[3]Output_PushPull;", "[0].RW.I32.port2/line2.NI.Line.Direction", "DIO line direction", "Line signal flow direction through the module, relative to the front I/O connector. This property is only used when the NI.ChannelEnable for this line is set to true. Changes to this property take effect after running the NI.ChannelConfigurationUpdate command."], "Child Tag"="Physical Channel/port2/line2/Properties/NI.Line.Direction", "Item Indent"=3, "Child Only?"=FALSE, "Glyph Index"=9}, {"Left Cell String"="NI.Line.Enable", "Child Text"=["False", "Read/Write", "Bool", "", "", "", "[0].RW.Bool.port2/line2.NI.Line.Enable", "DIO line output enable", "DIO output enable for one line. When a line is enabled, the input and output buffers for the front I/O connector and the rear I/O connector of the line are configured based on the NI.Line.Direction property. When a line is not enabled, the buffers for both the front I/O connector and the rear I/O connector are configured as inputs. Changes to this property take effect after running the NI.ChannelConfigurationUpdate command."], "Child Tag"="Physical Channel/port2/line2/Properties/NI.Line.Enable", "Item Indent"=3, "Child Only?"=FALSE, "Glyph Index"=9}, {"Left Cell String"="SLSC-12001-030EE1BC-Mod8/port2/line3", "Child Text"=[], "Child Tag"="Physical Channel/port2/line3", "Item Indent"=1, "Child Only?"=FALSE, "Glyph Index"=31}, {"Left Cell String"="Commands", "Child Text"=[], "Child Tag"="Physical Channel/port2/line3/Commands", "Item Indent"=2, "Child Only?"=FALSE, "Glyph Index"=35}, {"Left Cell String"="Properties", "Child Text"=[], "Child Tag"="Physical Channel/port2/line3/Properties", "Item Indent"=2, "Child Only?"=FALSE, "Glyph Index"=36}, {"Left Cell String"="NI.Line.Index", "Child Text"=["13", "Read Only", "U32", "", "", "", "[19].R.U32.port2/line3.NI.Line.Index", "Overall index of this DIO line in the module", "This is the index of this DIO line for the aggregate module properties: NI.FrontInputBufferState, NI.RearInputBufferState, and NI.TestModeValue."], "Child Tag"="Physical Channel/port2/line3/Properties/NI.Line.Index", "Item Indent"=3, "Child Only?"=FALSE, "Glyph Index"=8}, {"Left Cell String"="NI.Line.Direction", "Child Text"=["[0]Input", "Read/Write", "I32", "Enum", "NI.Line.Direction", "[0]Input;[1]Output_Source;[2]Output_Sink;[3]Output_PushPull;", "[0].RW.I32.port2/line3.NI.Line.Direction", "DIO line direction", "Line signal flow direction through the module, relative to the front I/O connector. This property is only used when the NI.ChannelEnable for this line is set to true. Changes to this property take effect after running the NI.ChannelConfigurationUpdate command."], "Child Tag"="Physical Channel/port2/line3/Properties/NI.Line.Direction", "Item Indent"=3, "Child Only?"=FALSE, "Glyph Index"=9}, {"Left Cell String"="NI.Line.Enable", "Child Text"=["False", "Read/Write", "Bool", "", "", "", "[0].RW.Bool.port2/line3.NI.Line.Enable", "DIO line output enable", "DIO output enable for one line. When a line is enabled, the input and output buffers for the front I/O connector and the rear I/O connector of the line are configured based on the NI.Line.Direction property. When a line is not enabled, the buffers for both the front I/O connector and the rear I/O connector are configured as inputs. Changes to this property take effect after running the NI.ChannelConfigurationUpdate command."], "Child Tag"="Physical Channel/port2/line3/Properties/NI.Line.Enable", "Item Indent"=3, "Child Only?"=FALSE, "Glyph Index"=9}, {"Left Cell String"="SLSC-12001-030EE1BC-Mod8/port2/line4", "Child Text"=[], "Child Tag"="Physical Channel/port2/line4", "Item Indent"=1, "Child Only?"=FALSE, "Glyph Index"=31}, {"Left Cell String"="Commands", "Child Text"=[], "Child Tag"="Physical Channel/port2/line4/Commands", "Item Indent"=2, "Child Only?"=FALSE, "Glyph Index"=35}, {"Left Cell String"="Properties", "Child Text"=[], "Child Tag"="Physical Channel/port2/line4/Properties", "Item Indent"=2, "Child Only?"=FALSE, "Glyph Index"=36}, {"Left Cell String"="NI.Line.Index", "Child Text"=["14", "Read Only", "U32", "", "", "", "[20].R.U32.port2/line4.NI.Line.Index", "Overall index of this DIO line in the module", "This is the index of this DIO line for the aggregate module properties: NI.FrontInputBufferState, NI.RearInputBufferState, and NI.TestModeValue."], "Child Tag"="Physical Channel/port2/line4/Properties/NI.Line.Index", "Item Indent"=3, "Child Only?"=FALSE, "Glyph Index"=8}, {"Left Cell String"="NI.Line.Direction", "Child Text"=["[0]Input", "Read/Write", "I32", "Enum", "NI.Line.Direction", "[0]Input;[1]Output_Source;[2]Output_Sink;[3]Output_PushPull;", "[0].RW.I32.port2/line4.NI.Line.Direction", "DIO line direction", "Line signal flow direction through the module, relative to the front I/O connector. This property is only used when the NI.ChannelEnable for this line is set to true. Changes to this property take effect after running the NI.ChannelConfigurationUpdate command."], "Child Tag"="Physical Channel/port2/line4/Properties/NI.Line.Direction", "Item Indent"=3, "Child Only?"=FALSE, "Glyph Index"=9}, {"Left Cell String"="NI.Line.Enable", "Child Text"=["False", "Read/Write", "Bool", "", "", "", "[0].RW.Bool.port2/line4.NI.Line.Enable", "DIO line output enable", "DIO output enable for one line. When a line is enabled, the input and output buffers for the front I/O connector and the rear I/O connector of the line are configured based on the NI.Line.Direction property. When a line is not enabled, the buffers for both the front I/O connector and the rear I/O connector are configured as inputs. Changes to this property take effect after running the NI.ChannelConfigurationUpdate command."], "Child Tag"="Physical Channel/port2/line4/Properties/NI.Line.Enable", "Item Indent"=3, "Child Only?"=FALSE, "Glyph Index"=9}, {"Left Cell String"="SLSC-12001-030EE1BC-Mod8/port2/line5", "Child Text"=[], "Child Tag"="Physical Channel/port2/line5", "Item Indent"=1, "Child Only?"=FALSE, "Glyph Index"=31}, {"Left Cell String"="Commands", "Child Text"=[], "Child Tag"="Physical Channel/port2/line5/Commands", "Item Indent"=2, "Child Only?"=FALSE, "Glyph Index"=35}, {"Left Cell String"="Properties", "Child Text"=[], "Child Tag"="Physical Channel/port2/line5/Properties", "Item Indent"=2, "Child Only?"=FALSE, "Glyph Index"=36}, {"Left Cell String"="NI.Line.Index", "Child Text"=["15", "Read Only", "U32", "", "", "", "[21].R.U32.port2/line5.NI.Line.Index", "Overall index of this DIO line in the module", "This is the index of this DIO line for the aggregate module properties: NI.FrontInputBufferState, NI.RearInputBufferState, and NI.TestModeValue."], "Child Tag"="Physical Channel/port2/line5/Properties/NI.Line.Index", "Item Indent"=3, "Child Only?"=FALSE, "Glyph Index"=8}, {"Left Cell String"="NI.Line.Direction", "Child Text"=["[0]Input", "Read/Write", "I32", "Enum", "NI.Line.Direction", "[0]Input;[1]Output_Source;[2]Output_Sink;[3]Output_PushPull;", "[0].RW.I32.port2/line5.NI.Line.Direction", "DIO line direction", "Line signal flow direction through the module, relative to the front I/O connector. This property is only used when the NI.ChannelEnable for this line is set to true. Changes to this property take effect after running the NI.ChannelConfigurationUpdate command."], "Child Tag"="Physical Channel/port2/line5/Properties/NI.Line.Direction", "Item Indent"=3, "Child Only?"=FALSE, "Glyph Index"=9}, {"Left Cell String"="NI.Line.Enable", "Child Text"=["False", "Read/Write", "Bool", "", "", "", "[0].RW.Bool.port2/line5.NI.Line.Enable", "DIO line output enable", "DIO output enable for one line. When a line is enabled, the input and output buffers for the front I/O connector and the rear I/O connector of the line are configured based on the NI.Line.Direction property. When a line is not enabled, the buffers for both the front I/O connector and the rear I/O connector are configured as inputs. Changes to this property take effect after running the NI.ChannelConfigurationUpdate command."], "Child Tag"="Physical Channel/port2/line5/Properties/NI.Line.Enable", "Item Indent"=3, "Child Only?"=FALSE, "Glyph Index"=9}, {"Left Cell String"="SLSC-12001-030EE1BC-Mod8/port2/line6", "Child Text"=[], "Child Tag"="Physical Channel/port2/line6", "Item Indent"=1, "Child Only?"=FALSE, "Glyph Index"=31}, {"Left Cell String"="Commands", "Child Text"=[], "Child Tag"="Physical Channel/port2/line6/Commands", "Item Indent"=2, "Child Only?"=FALSE, "Glyph Index"=35}, {"Left Cell String"="Properties", "Child Text"=[], "Child Tag"="Physical Channel/port2/line6/Properties", "Item Indent"=2, "Child Only?"=FALSE, "Glyph Index"=36}, {"Left Cell String"="NI.Line.Index", "Child Text"=["16", "Read Only", "U32", "", "", "", "[22].R.U32.port2/line6.NI.Line.Index", "Overall index of this DIO line in the module", "This is the index of this DIO line for the aggregate module properties: NI.FrontInputBufferState, NI.RearInputBufferState, and NI.TestModeValue."], "Child Tag"="Physical Channel/port2/line6/Properties/NI.Line.Index", "Item Indent"=3, "Child Only?"=FALSE, "Glyph Index"=8}, {"Left Cell String"="NI.Line.Direction", "Child Text"=["[0]Input", "Read/Write", "I32", "Enum", "NI.Line.Direction", "[0]Input;[1]Output_Source;[2]Output_Sink;[3]Output_PushPull;", "[0].RW.I32.port2/line6.NI.Line.Direction", "DIO line direction", "Line signal flow direction through the module, relative to the front I/O connector. This property is only used when the NI.ChannelEnable for this line is set to true. Changes to this property take effect after running the NI.ChannelConfigurationUpdate command."], "Child Tag"="Physical Channel/port2/line6/Properties/NI.Line.Direction", "Item Indent"=3, "Child Only?"=FALSE, "Glyph Index"=9}, {"Left Cell String"="NI.Line.Enable", "Child Text"=["False", "Read/Write", "Bool", "", "", "", "[0].RW.Bool.port2/line6.NI.Line.Enable", "DIO line output enable", "DIO output enable for one line. When a line is enabled, the input and output buffers for the front I/O connector and the rear I/O connector of the line are configured based on the NI.Line.Direction property. When a line is not enabled, the buffers for both the front I/O connector and the rear I/O connector are configured as inputs. Changes to this property take effect after running the NI.ChannelConfigurationUpdate command."], "Child Tag"="Physical Channel/port2/line6/Properties/NI.Line.Enable", "Item Indent"=3, "Child Only?"=FALSE, "Glyph Index"=9}, {"Left Cell String"="SLSC-12001-030EE1BC-Mod8/port2/line7", "Child Text"=[], "Child Tag"="Physical Channel/port2/line7", "Item Indent"=1, "Child Only?"=FALSE, "Glyph Index"=31}, {"Left Cell String"="Commands", "Child Text"=[], "Child Tag"="Physical Channel/port2/line7/Commands", "Item Indent"=2, "Child Only?"=FALSE, "Glyph Index"=35}, {"Left Cell String"="Properties", "Child Text"=[], "Child Tag"="Physical Channel/port2/line7/Properties", "Item Indent"=2, "Child Only?"=FALSE, "Glyph Index"=36}, {"Left Cell String"="NI.Line.Index", "Child Text"=["17", "Read Only", "U32", "", "", "", "[23].R.U32.port2/line7.NI.Line.Index", "Overall index of this DIO line in the module", "This is the index of this DIO line for the aggregate module properties: NI.FrontInputBufferState, NI.RearInputBufferState, and NI.TestModeValue."], "Child Tag"="Physical Channel/port2/line7/Properties/NI.Line.Index", "Item Indent"=3, "Child Only?"=FALSE, "Glyph Index"=8}, {"Left Cell String"="NI.Line.Direction", "Child Text"=["[0]Input", "Read/Write", "I32", "Enum", "NI.Line.Direction", "[0]Input;[1]Output_Source;[2]Output_Sink;[3]Output_PushPull;", "[0].RW.I32.port2/line7.NI.Line.Direction", "DIO line direction", "Line signal flow direction through the module, relative to the front I/O connector. This property is only used when the NI.ChannelEnable for this line is set to true. Changes to this property take effect after running the NI.ChannelConfigurationUpdate command."], "Child Tag"="Physical Channel/port2/line7/Properties/NI.Line.Direction", "Item Indent"=3, "Child Only?"=FALSE, "Glyph Index"=9}, {"Left Cell String"="NI.Line.Enable", "Child Text"=["False", "Read/Write", "Bool", "", "", "", "[0].RW.Bool.port2/line7.NI.Line.Enable", "DIO line output enable", "DIO output enable for one line. When a line is enabled, the input and output buffers for the front I/O connector and the rear I/O connector of the line are configured based on the NI.Line.Direction property. When a line is not enabled, the buffers for both the front I/O connector and the rear I/O connector are configured as inputs. Changes to this property take effect after running the NI.ChannelConfigurationUpdate command."], "Child Tag"="Physical Channel/port2/line7/Properties/NI.Line.Enable", "Item Indent"=3, "Child Only?"=FALSE, "Glyph Index"=9}, {"Left Cell String"="SLSC-12001-030EE1BC-Mod8/port3/line0", "Child Text"=[], "Child Tag"="Physical Channel/port3/line0", "Item Indent"=1, "Child Only?"=FALSE, "Glyph Index"=31}, {"Left Cell String"="Commands", "Child Text"=[], "Child Tag"="Physical Channel/port3/line0/Commands", "Item Indent"=2, "Child Only?"=FALSE, "Glyph Index"=35}, {"Left Cell String"="Properties", "Child Text"=[], "Child Tag"="Physical Channel/port3/line0/Properties", "Item Indent"=2, "Child Only?"=FALSE, "Glyph Index"=36}, {"Left Cell String"="NI.Line.Index", "Child Text"=["18", "Read Only", "U32", "", "", "", "[24].R.U32.port3/line0.NI.Line.Index", "Overall index of this DIO line in the module", "This is the index of this DIO line for the aggregate module properties: NI.FrontInputBufferState, NI.RearInputBufferState, and NI.TestModeValue."], "Child Tag"="Physical Channel/port3/line0/Properties/NI.Line.Index", "Item Indent"=3, "Child Only?"=FALSE, "Glyph Index"=8}, {"Left Cell String"="NI.Line.Direction", "Child Text"=["[0]Input", "Read/Write", "I32", "Enum", "NI.Line.Direction", "[0]Input;[1]Output_Source;[2]Output_Sink;[3]Output_PushPull;", "[0].RW.I32.port3/line0.NI.Line.Direction", "DIO line direction", "Line signal flow direction through the module, relative to the front I/O connector. This property is only used when the NI.ChannelEnable for this line is set to true. Changes to this property take effect after running the NI.ChannelConfigurationUpdate command."], "Child Tag"="Physical Channel/port3/line0/Properties/NI.Line.Direction", "Item Indent"=3, "Child Only?"=FALSE, "Glyph Index"=9}, {"Left Cell String"="NI.Line.Enable", "Child Text"=["False", "Read/Write", "Bool", "", "", "", "[0].RW.Bool.port3/line0.NI.Line.Enable", "DIO line output enable", "DIO output enable for one line. When a line is enabled, the input and output buffers for the front I/O connector and the rear I/O connector of the line are configured based on the NI.Line.Direction property. When a line is not enabled, the buffers for both the front I/O connector and the rear I/O connector are configured as inputs. Changes to this property take effect after running the NI.ChannelConfigurationUpdate command."], "Child Tag"="Physical Channel/port3/line0/Properties/NI.Line.Enable", "Item Indent"=3, "Child Only?"=FALSE, "Glyph Index"=9}, {"Left Cell String"="SLSC-12001-030EE1BC-Mod8/port3/line1", "Child Text"=[], "Child Tag"="Physical Channel/port3/line1", "Item Indent"=1, "Child Only?"=FALSE, "Glyph Index"=31}, {"Left Cell String"="Commands", "Child Text"=[], "Child Tag"="Physical Channel/port3/line1/Commands", "Item Indent"=2, "Child Only?"=FALSE, "Glyph Index"=35}, {"Left Cell String"="Properties", "Child Text"=[], "Child Tag"="Physical Channel/port3/line1/Properties", "Item Indent"=2, "Child Only?"=FALSE, "Glyph Index"=36}, {"Left Cell String"="NI.Line.Index", "Child Text"=["19", "Read Only", "U32", "", "", "", "[25].R.U32.port3/line1.NI.Line.Index", "Overall index of this DIO line in the module", "This is the index of this DIO line for the aggregate module properties: NI.FrontInputBufferState, NI.RearInputBufferState, and NI.TestModeValue."], "Child Tag"="Physical Channel/port3/line1/Properties/NI.Line.Index", "Item Indent"=3, "Child Only?"=FALSE, "Glyph Index"=8}, {"Left Cell String"="NI.Line.Direction", "Child Text"=["[0]Input", "Read/Write", "I32", "Enum", "NI.Line.Direction", "[0]Input;[1]Output_Source;[2]Output_Sink;[3]Output_PushPull;", "[0].RW.I32.port3/line1.NI.Line.Direction", "DIO line direction", "Line signal flow direction through the module, relative to the front I/O connector. This property is only used when the NI.ChannelEnable for this line is set to true. Changes to this property take effect after running the NI.ChannelConfigurationUpdate command."], "Child Tag"="Physical Channel/port3/line1/Properties/NI.Line.Direction", "Item Indent"=3, "Child Only?"=FALSE, "Glyph Index"=9}, {"Left Cell String"="NI.Line.Enable", "Child Text"=["False", "Read/Write", "Bool", "", "", "", "[0].RW.Bool.port3/line1.NI.Line.Enable", "DIO line output enable", "DIO output enable for one line. When a line is enabled, the input and output buffers for the front I/O connector and the rear I/O connector of the line are configured based on the NI.Line.Direction property. When a line is not enabled, the buffers for both the front I/O connector and the rear I/O connector are configured as inputs. Changes to this property take effect after running the NI.ChannelConfigurationUpdate command."], "Child Tag"="Physical Channel/port3/line1/Properties/NI.Line.Enable", "Item Indent"=3, "Child Only?"=FALSE, "Glyph Index"=9}, {"Left Cell String"="SLSC-12001-030EE1BC-Mod8/port3/line2", "Child Text"=[], "Child Tag"="Physical Channel/port3/line2", "Item Indent"=1, "Child Only?"=FALSE, "Glyph Index"=31}, {"Left Cell String"="Commands", "Child Text"=[], "Child Tag"="Physical Channel/port3/line2/Commands", "Item Indent"=2, "Child Only?"=FALSE, "Glyph Index"=35}, {"Left Cell String"="Properties", "Child Text"=[], "Child Tag"="Physical Channel/port3/line2/Properties", "Item Indent"=2, "Child Only?"=FALSE, "Glyph Index"=36}, {"Left Cell String"="NI.Line.Index", "Child Text"=["1A", "Read Only", "U32", "", "", "", "[26].R.U32.port3/line2.NI.Line.Index", "Overall index of this DIO line in the module", "This is the index of this DIO line for the aggregate module properties: NI.FrontInputBufferState, NI.RearInputBufferState, and NI.TestModeValue."], "Child Tag"="Physical Channel/port3/line2/Properties/NI.Line.Index", "Item Indent"=3, "Child Only?"=FALSE, "Glyph Index"=8}, {"Left Cell String"="NI.Line.Direction", "Child Text"=["[0]Input", "Read/Write", "I32", "Enum", "NI.Line.Direction", "[0]Input;[1]Output_Source;[2]Output_Sink;[3]Output_PushPull;", "[0].RW.I32.port3/line2.NI.Line.Direction", "DIO line direction", "Line signal flow direction through the module, relative to the front I/O connector. This property is only used when the NI.ChannelEnable for this line is set to true. Changes to this property take effect after running the NI.ChannelConfigurationUpdate command."], "Child Tag"="Physical Channel/port3/line2/Properties/NI.Line.Direction", "Item Indent"=3, "Child Only?"=FALSE, "Glyph Index"=9}, {"Left Cell String"="NI.Line.Enable", "Child Text"=["False", "Read/Write", "Bool", "", "", "", "[0].RW.Bool.port3/line2.NI.Line.Enable", "DIO line output enable", "DIO output enable for one line. When a line is enabled, the input and output buffers for the front I/O connector and the rear I/O connector of the line are configured based on the NI.Line.Direction property. When a line is not enabled, the buffers for both the front I/O connector and the rear I/O connector are configured as inputs. Changes to this property take effect after running the NI.ChannelConfigurationUpdate command."], "Child Tag"="Physical Channel/port3/line2/Properties/NI.Line.Enable", "Item Indent"=3, "Child Only?"=FALSE, "Glyph Index"=9}, {"Left Cell String"="SLSC-12001-030EE1BC-Mod8/port3/line3", "Child Text"=[], "Child Tag"="Physical Channel/port3/line3", "Item Indent"=1, "Child Only?"=FALSE, "Glyph Index"=31}, {"Left Cell String"="Commands", "Child Text"=[], "Child Tag"="Physical Channel/port3/line3/Commands", "Item Indent"=2, "Child Only?"=FALSE, "Glyph Index"=35}, {"Left Cell String"="Properties", "Child Text"=[], "Child Tag"="Physical Channel/port3/line3/Properties", "Item Indent"=2, "Child Only?"=FALSE, "Glyph Index"=36}, {"Left Cell String"="NI.Line.Index", "Child Text"=["1B", "Read Only", "U32", "", "", "", "[27].R.U32.port3/line3.NI.Line.Index", "Overall index of this DIO line in the module", "This is the index of this DIO line for the aggregate module properties: NI.FrontInputBufferState, NI.RearInputBufferState, and NI.TestModeValue."], "Child Tag"="Physical Channel/port3/line3/Properties/NI.Line.Index", "Item Indent"=3, "Child Only?"=FALSE, "Glyph Index"=8}, {"Left Cell String"="NI.Line.Direction", "Child Text"=["[0]Input", "Read/Write", "I32", "Enum", "NI.Line.Direction", "[0]Input;[1]Output_Source;[2]Output_Sink;[3]Output_PushPull;", "[0].RW.I32.port3/line3.NI.Line.Direction", "DIO line direction", "Line signal flow direction through the module, relative to the front I/O connector. This property is only used when the NI.ChannelEnable for this line is set to true. Changes to this property take effect after running the NI.ChannelConfigurationUpdate command."], "Child Tag"="Physical Channel/port3/line3/Properties/NI.Line.Direction", "Item Indent"=3, "Child Only?"=FALSE, "Glyph Index"=9}, {"Left Cell String"="NI.Line.Enable", "Child Text"=["False", "Read/Write", "Bool", "", "", "", "[0].RW.Bool.port3/line3.NI.Line.Enable", "DIO line output enable", "DIO output enable for one line. When a line is enabled, the input and output buffers for the front I/O connector and the rear I/O connector of the line are configured based on the NI.Line.Direction property. When a line is not enabled, the buffers for both the front I/O connector and the rear I/O connector are configured as inputs. Changes to this property take effect after running the NI.ChannelConfigurationUpdate command."], "Child Tag"="Physical Channel/port3/line3/Properties/NI.Line.Enable", "Item Indent"=3, "Child Only?"=FALSE, "Glyph Index"=9}, {"Left Cell String"="SLSC-12001-030EE1BC-Mod8/port3/line4", "Child Text"=[], "Child Tag"="Physical Channel/port3/line4", "Item Indent"=1, "Child Only?"=FALSE, "Glyph Index"=31}, {"Left Cell String"="Commands", "Child Text"=[], "Child Tag"="Physical Channel/port3/line4/Commands", "Item Indent"=2, "Child Only?"=FALSE, "Glyph Index"=35}, {"Left Cell String"="Properties", "Child Text"=[], "Child Tag"="Physical Channel/port3/line4/Properties", "Item Indent"=2, "Child Only?"=FALSE, "Glyph Index"=36}, {"Left Cell String"="NI.Line.Index", "Child Text"=["1C", "Read Only", "U32", "", "", "", "[28].R.U32.port3/line4.NI.Line.Index", "Overall index of this DIO line in the module", "This is the index of this DIO line for the aggregate module properties: NI.FrontInputBufferState, NI.RearInputBufferState, and NI.TestModeValue."], "Child Tag"="Physical Channel/port3/line4/Properties/NI.Line.Index", "Item Indent"=3, "Child Only?"=FALSE, "Glyph Index"=8}, {"Left Cell String"="NI.Line.Direction", "Child Text"=["[0]Input", "Read/Write", "I32", "Enum", "NI.Line.Direction", "[0]Input;[1]Output_Source;[2]Output_Sink;[3]Output_PushPull;", "[0].RW.I32.port3/line4.NI.Line.Direction", "DIO line direction", "Line signal flow direction through the module, relative to the front I/O connector. This property is only used when the NI.ChannelEnable for this line is set to true. Changes to this property take effect after running the NI.ChannelConfigurationUpdate command."], "Child Tag"="Physical Channel/port3/line4/Properties/NI.Line.Direction", "Item Indent"=3, "Child Only?"=FALSE, "Glyph Index"=9}, {"Left Cell String"="NI.Line.Enable", "Child Text"=["False", "Read/Write", "Bool", "", "", "", "[0].RW.Bool.port3/line4.NI.Line.Enable", "DIO line output enable", "DIO output enable for one line. When a line is enabled, the input and output buffers for the front I/O connector and the rear I/O connector of the line are configured based on the NI.Line.Direction property. When a line is not enabled, the buffers for both the front I/O connector and the rear I/O connector are configured as inputs. Changes to this property take effect after running the NI.ChannelConfigurationUpdate command."], "Child Tag"="Physical Channel/port3/line4/Properties/NI.Line.Enable", "Item Indent"=3, "Child Only?"=FALSE, "Glyph Index"=9}, {"Left Cell String"="SLSC-12001-030EE1BC-Mod8/port3/line5", "Child Text"=[], "Child Tag"="Physical Channel/port3/line5", "Item Indent"=1, "Child Only?"=FALSE, "Glyph Index"=31}, {"Left Cell String"="Commands", "Child Text"=[], "Child Tag"="Physical Channel/port3/line5/Commands", "Item Indent"=2, "Child Only?"=FALSE, "Glyph Index"=35}, {"Left Cell String"="Properties", "Child Text"=[], "Child Tag"="Physical Channel/port3/line5/Properties", "Item Indent"=2, "Child Only?"=FALSE, "Glyph Index"=36}, {"Left Cell String"="NI.Line.Index", "Child Text"=["1D", "Read Only", "U32", "", "", "", "[29].R.U32.port3/line5.NI.Line.Index", "Overall index of this DIO line in the module", "This is the index of this DIO line for the aggregate module properties: NI.FrontInputBufferState, NI.RearInputBufferState, and NI.TestModeValue."], "Child Tag"="Physical Channel/port3/line5/Properties/NI.Line.Index", "Item Indent"=3, "Child Only?"=FALSE, "Glyph Index"=8}, {"Left Cell String"="NI.Line.Direction", "Child Text"=["[0]Input", "Read/Write", "I32", "Enum", "NI.Line.Direction", "[0]Input;[1]Output_Source;[2]Output_Sink;[3]Output_PushPull;", "[0].RW.I32.port3/line5.NI.Line.Direction", "DIO line direction", "Line signal flow direction through the module, relative to the front I/O connector. This property is only used when the NI.ChannelEnable for this line is set to true. Changes to this property take effect after running the NI.ChannelConfigurationUpdate command."], "Child Tag"="Physical Channel/port3/line5/Properties/NI.Line.Direction", "Item Indent"=3, "Child Only?"=FALSE, "Glyph Index"=9}, {"Left Cell String"="NI.Line.Enable", "Child Text"=["False", "Read/Write", "Bool", "", "", "", "[0].RW.Bool.port3/line5.NI.Line.Enable", "DIO line output enable", "DIO output enable for one line. When a line is enabled, the input and output buffers for the front I/O connector and the rear I/O connector of the line are configured based on the NI.Line.Direction property. When a line is not enabled, the buffers for both the front I/O connector and the rear I/O connector are configured as inputs. Changes to this property take effect after running the NI.ChannelConfigurationUpdate command."], "Child Tag"="Physical Channel/port3/line5/Properties/NI.Line.Enable", "Item Indent"=3, "Child Only?"=FALSE, "Glyph Index"=9}, {"Left Cell String"="SLSC-12001-030EE1BC-Mod8/port3/line6", "Child Text"=[], "Child Tag"="Physical Channel/port3/line6", "Item Indent"=1, "Child Only?"=FALSE, "Glyph Index"=31}, {"Left Cell String"="Commands", "Child Text"=[], "Child Tag"="Physical Channel/port3/line6/Commands", "Item Indent"=2, "Child Only?"=FALSE, "Glyph Index"=35}, {"Left Cell String"="Properties", "Child Text"=[], "Child Tag"="Physical Channel/port3/line6/Properties", "Item Indent"=2, "Child Only?"=FALSE, "Glyph Index"=36}, {"Left Cell String"="NI.Line.Index", "Child Text"=["1E", "Read Only", "U32", "", "", "", "[30].R.U32.port3/line6.NI.Line.Index", "Overall index of this DIO line in the module", "This is the index of this DIO line for the aggregate module properties: NI.FrontInputBufferState, NI.RearInputBufferState, and NI.TestModeValue."], "Child Tag"="Physical Channel/port3/line6/Properties/NI.Line.Index", "Item Indent"=3, "Child Only?"=FALSE, "Glyph Index"=8}, {"Left Cell String"="NI.Line.Direction", "Child Text"=["[0]Input", "Read/Write", "I32", "Enum", "NI.Line.Direction", "[0]Input;[1]Output_Source;[2]Output_Sink;[3]Output_PushPull;", "[0].RW.I32.port3/line6.NI.Line.Direction", "DIO line direction", "Line signal flow direction through the module, relative to the front I/O connector. This property is only used when the NI.ChannelEnable for this line is set to true. Changes to this property take effect after running the NI.ChannelConfigurationUpdate command."], "Child Tag"="Physical Channel/port3/line6/Properties/NI.Line.Direction", "Item Indent"=3, "Child Only?"=FALSE, "Glyph Index"=9}, {"Left Cell String"="NI.Line.Enable", "Child Text"=["False", "Read/Write", "Bool", "", "", "", "[0].RW.Bool.port3/line6.NI.Line.Enable", "DIO line output enable", "DIO output enable for one line. When a line is enabled, the input and output buffers for the front I/O connector and the rear I/O connector of the line are configured based on the NI.Line.Direction property. When a line is not enabled, the buffers for both the front I/O connector and the rear I/O connector are configured as inputs. Changes to this property take effect after running the NI.ChannelConfigurationUpdate command."], "Child Tag"="Physical Channel/port3/line6/Properties/NI.Line.Enable", "Item Indent"=3, "Child Only?"=FALSE, "Glyph Index"=9}, {"Left Cell String"="SLSC-12001-030EE1BC-Mod8/port3/line7", "Child Text"=[], "Child Tag"="Physical Channel/port3/line7", "Item Indent"=1, "Child Only?"=FALSE, "Glyph Index"=31}, {"Left Cell String"="Commands", "Child Text"=[], "Child Tag"="Physical Channel/port3/line7/Commands", "Item Indent"=2, "Child Only?"=FALSE, "Glyph Index"=35}, {"Left Cell String"="Properties", "Child Text"=[], "Child Tag"="Physical Channel/port3/line7/Properties", "Item Indent"=2, "Child Only?"=FALSE, "Glyph Index"=36}, {"Left Cell String"="NI.Line.Index", "Child Text"=["1F", "Read Only", "U32", "", "", "", "[31].R.U32.port3/line7.NI.Line.Index", "Overall index of this DIO line in the module", "This is the index of this DIO line for the aggregate module properties: NI.FrontInputBufferState, NI.RearInputBufferState, and NI.TestModeValue."], "Child Tag"="Physical Channel/port3/line7/Properties/NI.Line.Index", "Item Indent"=3, "Child Only?"=FALSE, "Glyph Index"=8}, {"Left Cell String"="NI.Line.Direction", "Child Text"=["[0]Input", "Read/Write", "I32", "Enum", "NI.Line.Direction", "[0]Input;[1]Output_Source;[2]Output_Sink;[3]Output_PushPull;", "[0].RW.I32.port3/line7.NI.Line.Direction", "DIO line direction", "Line signal flow direction through the module, relative to the front I/O connector. This property is only used when the NI.ChannelEnable for this line is set to true. Changes to this property take effect after running the NI.ChannelConfigurationUpdate command."], "Child Tag"="Physical Channel/port3/line7/Properties/NI.Line.Direction", "Item Indent"=3, "Child Only?"=FALSE, "Glyph Index"=9}, {"Left Cell String"="NI.Line.Enable", "Child Text"=["False", "Read/Write", "Bool", "", "", "", "[0].RW.Bool.port3/line7.NI.Line.Enable", "DIO line output enable", "DIO output enable for one line. When a line is enabled, the input and output buffers for the front I/O connector and the rear I/O connector of the line are configured based on the NI.Line.Direction property. When a line is not enabled, the buffers for both the front I/O connector and the rear I/O connector are configured as inputs. Changes to this property take effect after running the NI.ChannelConfigurationUpdate command."], "Child Tag"="Physical Channel/port3/line7/Properties/NI.Line.Enable", "Item Indent"=3, "Child Only?"=FALSE, "Glyph Index"=9}])   [LabVIEW 2017, in "SLSC Tree Control.lvlib"]
doc: "Creates a SLSC tree control based on the SLSC EDS datatype (Capabilities)."
uses:
  SLSC Tree Control.lvlib
  Ctrl/Enum.ctl
  Ctrl/EDSjsonStructure.ctl
  Ctrl/command.ctl
  Ctrl/PhysicalChannel.ctl
  Ctrl/Property.ctl
  Ctrl/Scale.ctl
  Ctrl/Register.ctl
  Ctrl/EnumValue.ctl
panel:
  out "Array 2":string[](array[string])
  out "Array":string[](array[string])
  in  "stop":bool
  out "Property tree 2":string[](array[string])
  in  "Property tree":string[](tree)
  # "not working\nregisterMap->registers->initialValue"
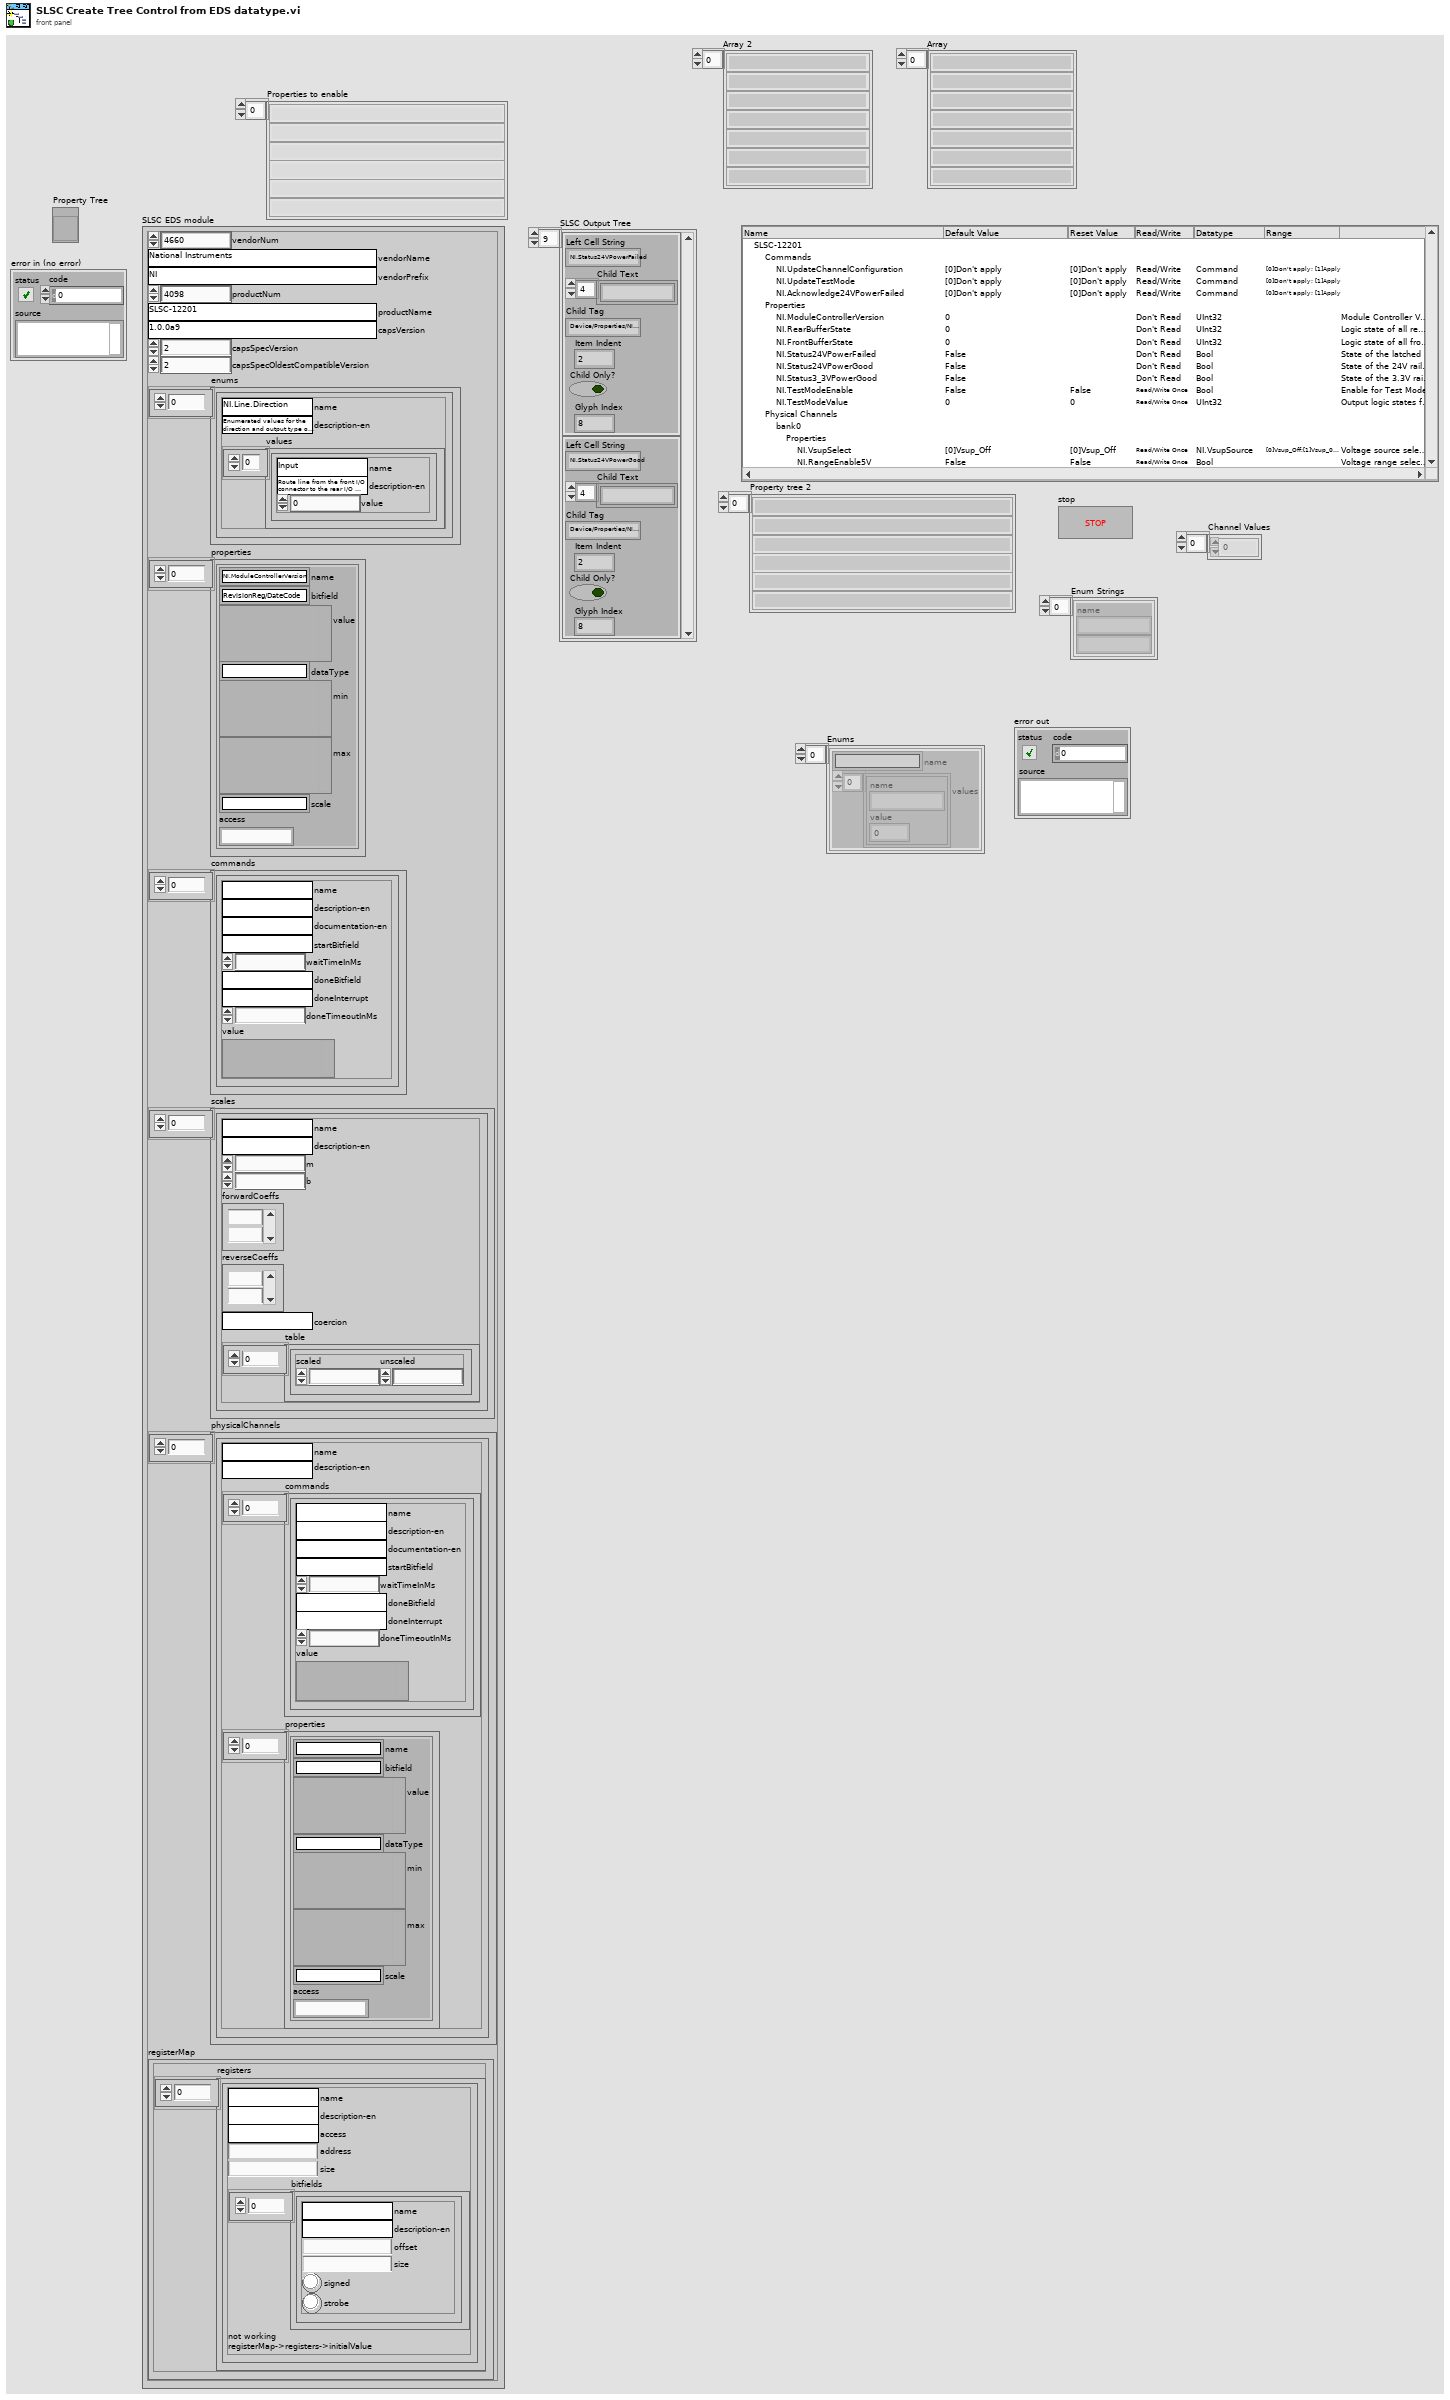
[diagram p1: front panel]
types:
  T1 = typedef "Enum.ctl" = cluster{"name":string, "values":T2[]}
  T2 = typedef "EnumValue.ctl" = cluster{"name":string, "value":i32}
  T3 = cluster{"Left Cell String":string, "Child Text":string[], "Child Tag":string, "Item Indent":i32, "Child Only?":bool, "Glyph Index":i32}[]
  T4 = typedef "EDSjsonStructure.ctl" = cluster{"vendorNum":u32, "vendorName":string, "vendorPrefix":string, "productNum":u32, "productName":string, "capsVersion":string, "capsSpecVersion":u32, "capsSpecOldestCompatibleVersion":u32, "enums":T5[], "properties":T6[], "commands":T7[], "scales":T8[], "physicalChannels":T9[], "registerMap":cluster{"registers":T10[]}}
  T5 = typedef "enum.ctl" = cluster{"name":string, "description-en":string, "values":cluster{"name":string, "description-en":string, "value":i32}[]}
  T6 = typedef "Property.ctl" = cluster{"name":string, "bitfield":string, "value":variant, "dataType":string, "min":variant, "max":variant, "scale":string, "access":string}
  T7 = typedef "command.ctl" = cluster{"name":string, "description-en":string, "documentation-en":string, "startBitfield":string, "waitTimeInMs":i32, "doneBitfield":string, "doneInterrupt":string, "doneTimeoutInMs":i32, "value":variant}
  T8 = typedef "scale.ctl" = cluster{"name":string, "description-en":string, "m":dbl, "b":dbl, "forwardCoeffs":dbl[], "reverseCoeffs":dbl[], "coercion":string, "table":cluster{"scaled":dbl, "unscaled":dbl}[]}
  T9 = typedef "PhysicalChannel.ctl" = cluster{"name":string, "description-en":string, "commands":T7[], "properties":T6[]}
  T10 = typedef "register.ctl" = cluster{"name":string, "description-en":string, "access":string, "address":u32, "size":u32, "bitfields":cluster{"name":string, "description-en":string, "offset":u32, "size":u32, "signed":bool, "strobe":bool}[]}
  T11 = typedef "imagedata.ctl" = cluster{"image type":i32, "image depth":i32, "image":u8[], "mask":u8[], "colors":u32[], "Rectangle":cluster{"left":i16, "top":i16, "right":i16, "bottom":i16}}
  T12 = cluster{"name":string, "string enums":string, "values":T2[]}[]
  T13 = cluster{"Left Cell String":string, "Child Text":string[], "Child Tag":string, "Item Indent":i32, "Child Only?":bool, "Glyph Index":i32, "offline value":variant}
  T14 = cluster{"Left Cell String":string, "Child Text":string[], "Child Tag":string, "Item Indent":i32, "Child Only?":bool, "Glyph Index":i32, "offline value":variant}[]
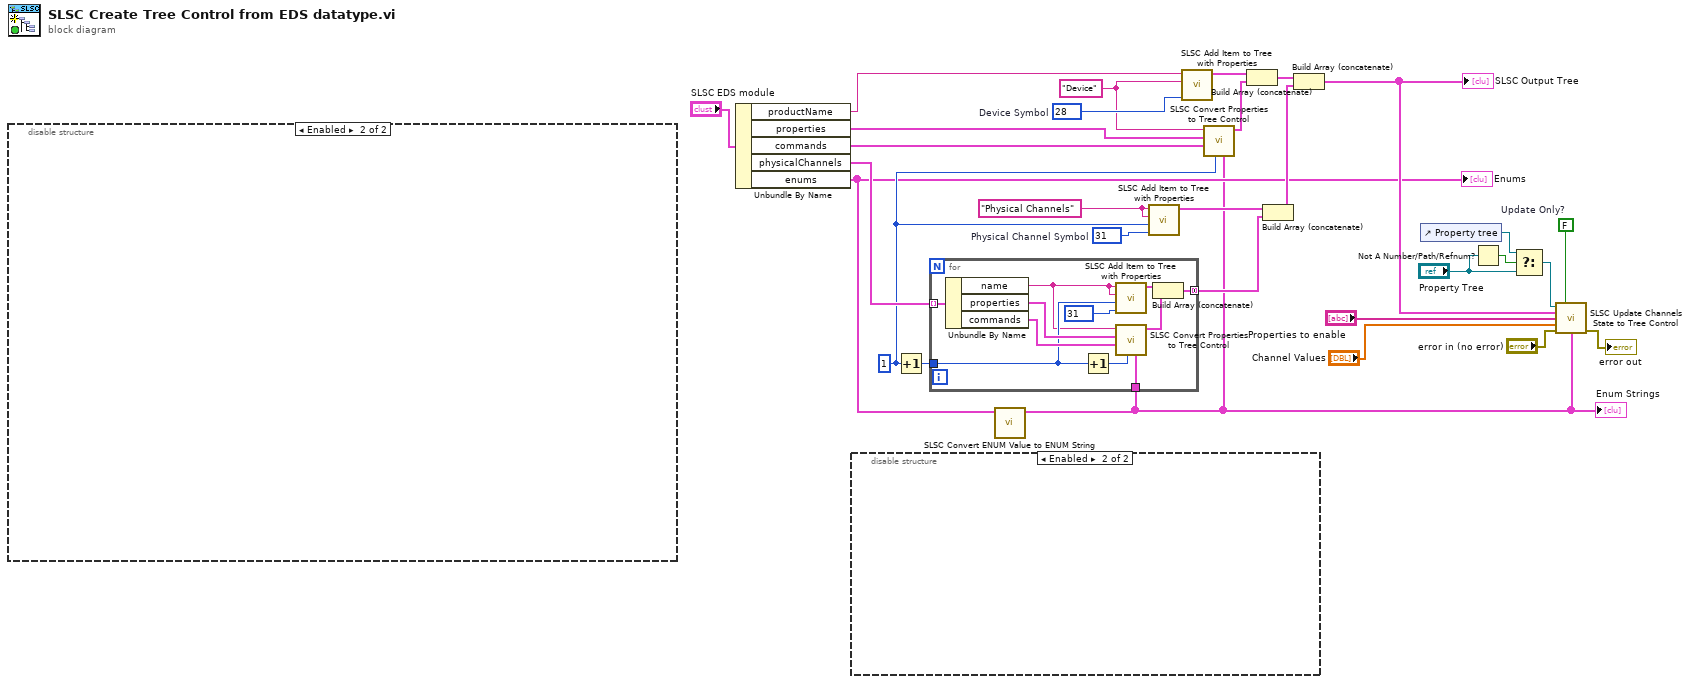
[diagram p0: block diagram]
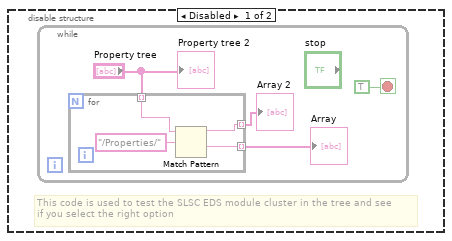
[diagram p2: hidden frame]
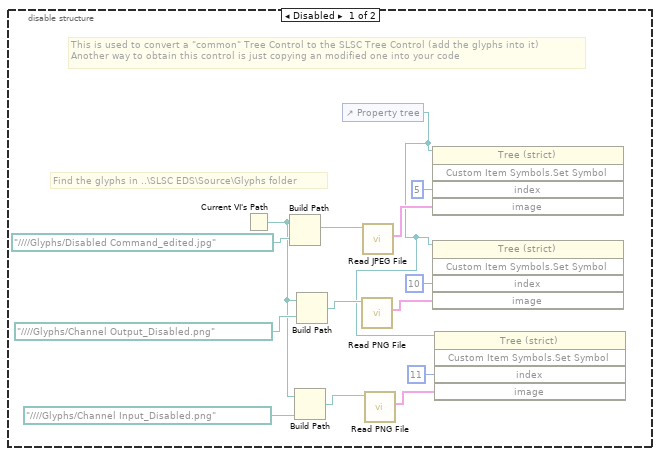
[diagram p3: hidden frame]
diagram:
  w3 = FALSE  # Update Only?
  w15 = 31  # Physical Channel Symbol
  w16 = "Physical Channels" ("Child Tag")
  w11 = 1 ("Item Indent")
  w28 = 28  # Device Symbol
  w21 = "Device" ("Child Tag")
  n1 = disable-structure shown="Enabled" {
    frame Disabled {
      # "Find the glyphs in ..\\SLSC EDS\\Source\\Glyphs folder"
      # "This is used to convert a \"common\" Tree Control to the SLSC Tree Control (add the glyphs into it)\nAnother way to obtain this control is just copying an modified one into your code"
      n2 = Current VI's Path() -> (path=w31:path)
      n3 = Build Path(base path=w31, name or relative path=path "../../../../Glyphs/Disabled Command_edited.jpg" ("path to PNG file")) -> (appended path=w38:path)
      n4 = Build Path(base path=w31, name or relative path=path "../../../../Glyphs/Channel Input_Disabled.png" ("path to PNG file")) -> (appended path=w30:path)
      n5 = Build Path(base path=w31, name or relative path=path "../../../../Glyphs/Channel Output_Disabled.png" ("path to PNG file")) -> (appended path=w36:path)
      n6 = control-ref of="Property tree"() -> (w34:refnum<vi>)
      n7 = call <vilib>:"Read PNG File.vi"("path to PNG file"=w36) -> ("image data"=w39:T11)  [unwired: 8 in, 2 out]
      n8 = call <vilib>:"Read JPEG File.vi"("path to JPEG file"=w38) -> ("image data"=w42:T11)  [unwired: 8 in, 2 out]
      n9 = call <vilib>:"Read PNG File.vi"("path to PNG file"=w30) -> ("image data"=w33:T11)  [unwired: 8 in, 2 out]
      n10 = invoke on="Invoke Node" class="Tree (strict)" method="Custom Item Symbols.Set Symbol"(reference=w34, "index"=5 ("Index"), "image"=w42) -> ()  [unwired: 2 in, 5 out]
      n11 = invoke on="Invoke Node" class="Tree (strict)" method="Custom Item Symbols.Set Symbol"(reference=w34, "index"=10 ("Index"), "image"=w39) -> ()  [unwired: 2 in, 5 out]
      n12 = invoke on="Invoke Node" class="Tree (strict)" method="Custom Item Symbols.Set Symbol"(reference=w34, "index"=11 ("Index"), "image"=w33) -> ()  [unwired: 2 in, 5 out]
    }
    frame Enabled {
    }
  }
  n13 = Unbundle By Name("SLSC EDS module") -> ("productName"=w27:string, "properties"=w23:T6[], "commands"=w24:T7[], "physicalChannels"=w20:T9[], "enums"=w4:T5[])
  "Enums" <- w4
  n14 = disable-structure shown="Enabled" {
    frame Disabled {
      # "This code is used to test the SLSC EDS module cluster in the tree and see\nif you select the right option"
      n15 = while {
        stop <- TRUE stop-if-true
        n16 = for {
          tunnel: "Property tree" -> [w50] mode=indexing
          tunnel: [w49] -> w45 mode=indexing
          tunnel: [w48] -> w44 mode=indexing
          n17 = Match Pattern(string=w50, regular expression="/Properties/") -> (before substring=w48:string, after substring=w49:string)  [unwired: 1 in, 2 out]
        }
        "Array" <- w45
        "Array 2" <- w44
        "Property tree 2" <- "Property tree"
      }
    }
    frame Enabled {
    }
  }
  n18 = Increment(x=w11) -> (x+1=w10:i32)
  n19 = call "SLSC Convert ENUM Value to ENUM String.vi"("enums"=w4) -> ("string enums"=w2:T12)  [unwired: 10 in]
  "Enum Strings" <- w2
  n20 = for {
    tunnel: w20 -> [w62] mode=indexing
    tunnel: w10 -> [w54]
    tunnel: [w56] -> w14 mode=concatenating
    tunnel: w2 -> [w52]
    n21 = Unbundle By Name(w62) -> ("name"=w53:string, "properties"=w59:T6[], "commands"=w58:T7[])
    n22 = Increment(x=w54) -> (x+1=w57:i32)
    n23 = call "SLSC Add Item to Tree with Properties.vi"("Glyph Index"=31, "Item indent"=w54, "Child Tag"=w53, "Left Cell String"=w53) -> ("Item"=w60:T13)  [unwired: 7 in]
    n24 = call "SLSC Convert Properties to Tree Control.vi"("string enums"=w52, "Item Indent"=w57, "Init Values"=w58, "properties"=w59, "Child Tag"=w53) -> ("Tree Items"=w61:T14)  [unwired: 6 in]
    n25 = Build Array (concatenate)(w60, w61) -> (w56:T14)
  }
  n26 = call "SLSC Add Item to Tree with Properties.vi"("Glyph Index"=w15, "Item indent"=w11, "Child Tag"=w16, "Left Cell String"=w16) -> ("Item"=w13:T13)  [unwired: 7 in]
  n27 = call "SLSC Add Item to Tree with Properties.vi"("Glyph Index"=w28, "Child Tag"=w21, "Left Cell String"=w27) -> ("Item"=w25:T13)  [unwired: 8 in]
  n28 = call "SLSC Convert Properties to Tree Control.vi"("string enums"=w2, "Item Indent"=w11, "Init Values"=w24, "properties"=w23, "Child Tag"=w21) -> ("Tree Items"=w22:T14)  [unwired: 6 in]
  n29 = Build Array (concatenate)(w25, w22) -> (w26:T14)
  n30 = Build Array (concatenate)(w13, w14) -> (w12:T14)
  n31 = Build Array (concatenate)(w26, w12) -> (w19:T14)
  "SLSC Output Tree" <- w19
  n32 = control-ref of="Property tree"() -> (w7:refnum<vi>)
  n33 = Not A Number/Path/Refnum?(number/path/refnum="Property Tree") -> (NaN/Path/Refnum?=w9:bool)
  n34 = Select(t=w7, s=w9, f="Property Tree") -> (s? t:f=w6:refnum<vi>)
  n35 = call "SLSC Update Channels State to Tree Control.vi"("Property tree"=w6, "Update Only?"=w3, "SLSC Output Tree"=w19, "Channels to \"enable\""="Properties to enable", "Channel Values"="Channel Values", "error in (no error)"="error in (no error)", "string enums"=w2) -> ("error out"=→"error out":errorcluster)  [unwired: 8 in]
